vi "Export.vi"(9 "warehosue database table":string[](array[string]), 10 "Path":path, 11 "connection in":T4) -> (3 "connection out":T4)   [LabVIEW 2017]
uses:
  <vilib>/addons/database/Connection.llb/Conn ObjectReference.ctl
  Control/item colum type.ctl
  Control/Produce colum type.ctl
  <vilib>/Utility/miscctls.llb/LVPointTypeDef.ctl
  <vilib>/Utility/miscctls.llb/LVRowAndColumnUnsignedTypeDef.ctl
  Control/State machine.ctl
  Control/Label data.ctl
  <vilib>/addons/database/Connection.llb/DB Tools Open Connec (Path).vi
  <vilib>/addons/_office/excel.llb/Excel Get Data ([str]).vi
  <vilib>/addons/database/Connection.llb/Conn Execute.vi
  <vilib>/addons/database/Recordset.llb/Rec Fetch Recordset Data (R).vi
  <vilib>/addons/database/Recordset.llb/Rec Destroy - Connection.vi
  <vilib>/addons/database/_DB Variant To Data/Database Variant To Data.xnode
  <vilib>/Utility/NIReport.llb/NI_report.lvclass
  <vilib>/addons/_office/NI_ReportGenerationToolkit.lvlib
  <vilib>/addons/database/NI_Database_API.lvlib
  <vilib>/Utility/NIReport.llb/Excel/NI_Excel.lvclass
panel:
  out "output cluster":T1
  in  "produce_data":T1
  out "reference":refnum<vi>[](array[refnum])
  in  "Print Mode 2":bool=TRUE
  out "IQA":string
  out "stock":string
  in  "Print Mode":bool=TRUE
  in  "Print":bool
  in  "Item No.(F8)":i32
  in  "item_data":T2
  out "item_data_name":string[](array[string])
  out "item_data_ctr":refnum<vi>[](array[refnum])
  out "ECODE":string
  out "PRODUCE_data_ctr":refnum<vi>[](array[refnum])
  out "PRODUCE_data_name":string[](array[string])
  out "File data":string[][](array[string])
  in  "Import data":T3 {"produce Date" format="%<%d/%m/%Y>T"}
  in  "Lot Maker (F9)":string
  in  "Location (F5)":string
  in  "Maker Code (F4)":string
  in  "BUTTON_ADD":bool
  in  "Quantity (F10)":string
  in  "Lot Size (F6)":string
  in  "Unit (F7)":string
  in  "Item Code (F3)":string
  in  "Part No (F2)":string(combo)
  in  "Barcode (F1)":string
  in  "Offset":string="0"
  in  "Length":string="0"
  in  "Maker":string(combo)
  in  "Part Name":string(combo)
  in  "Product":string(combo)
  out "Produce Date":timestamp format="%<%d/%m/%Y>T"
  out "produce Code":string caption="Produce Code"
  out "Table":string[][](table)
  # "PRODUCE EXMPORT"
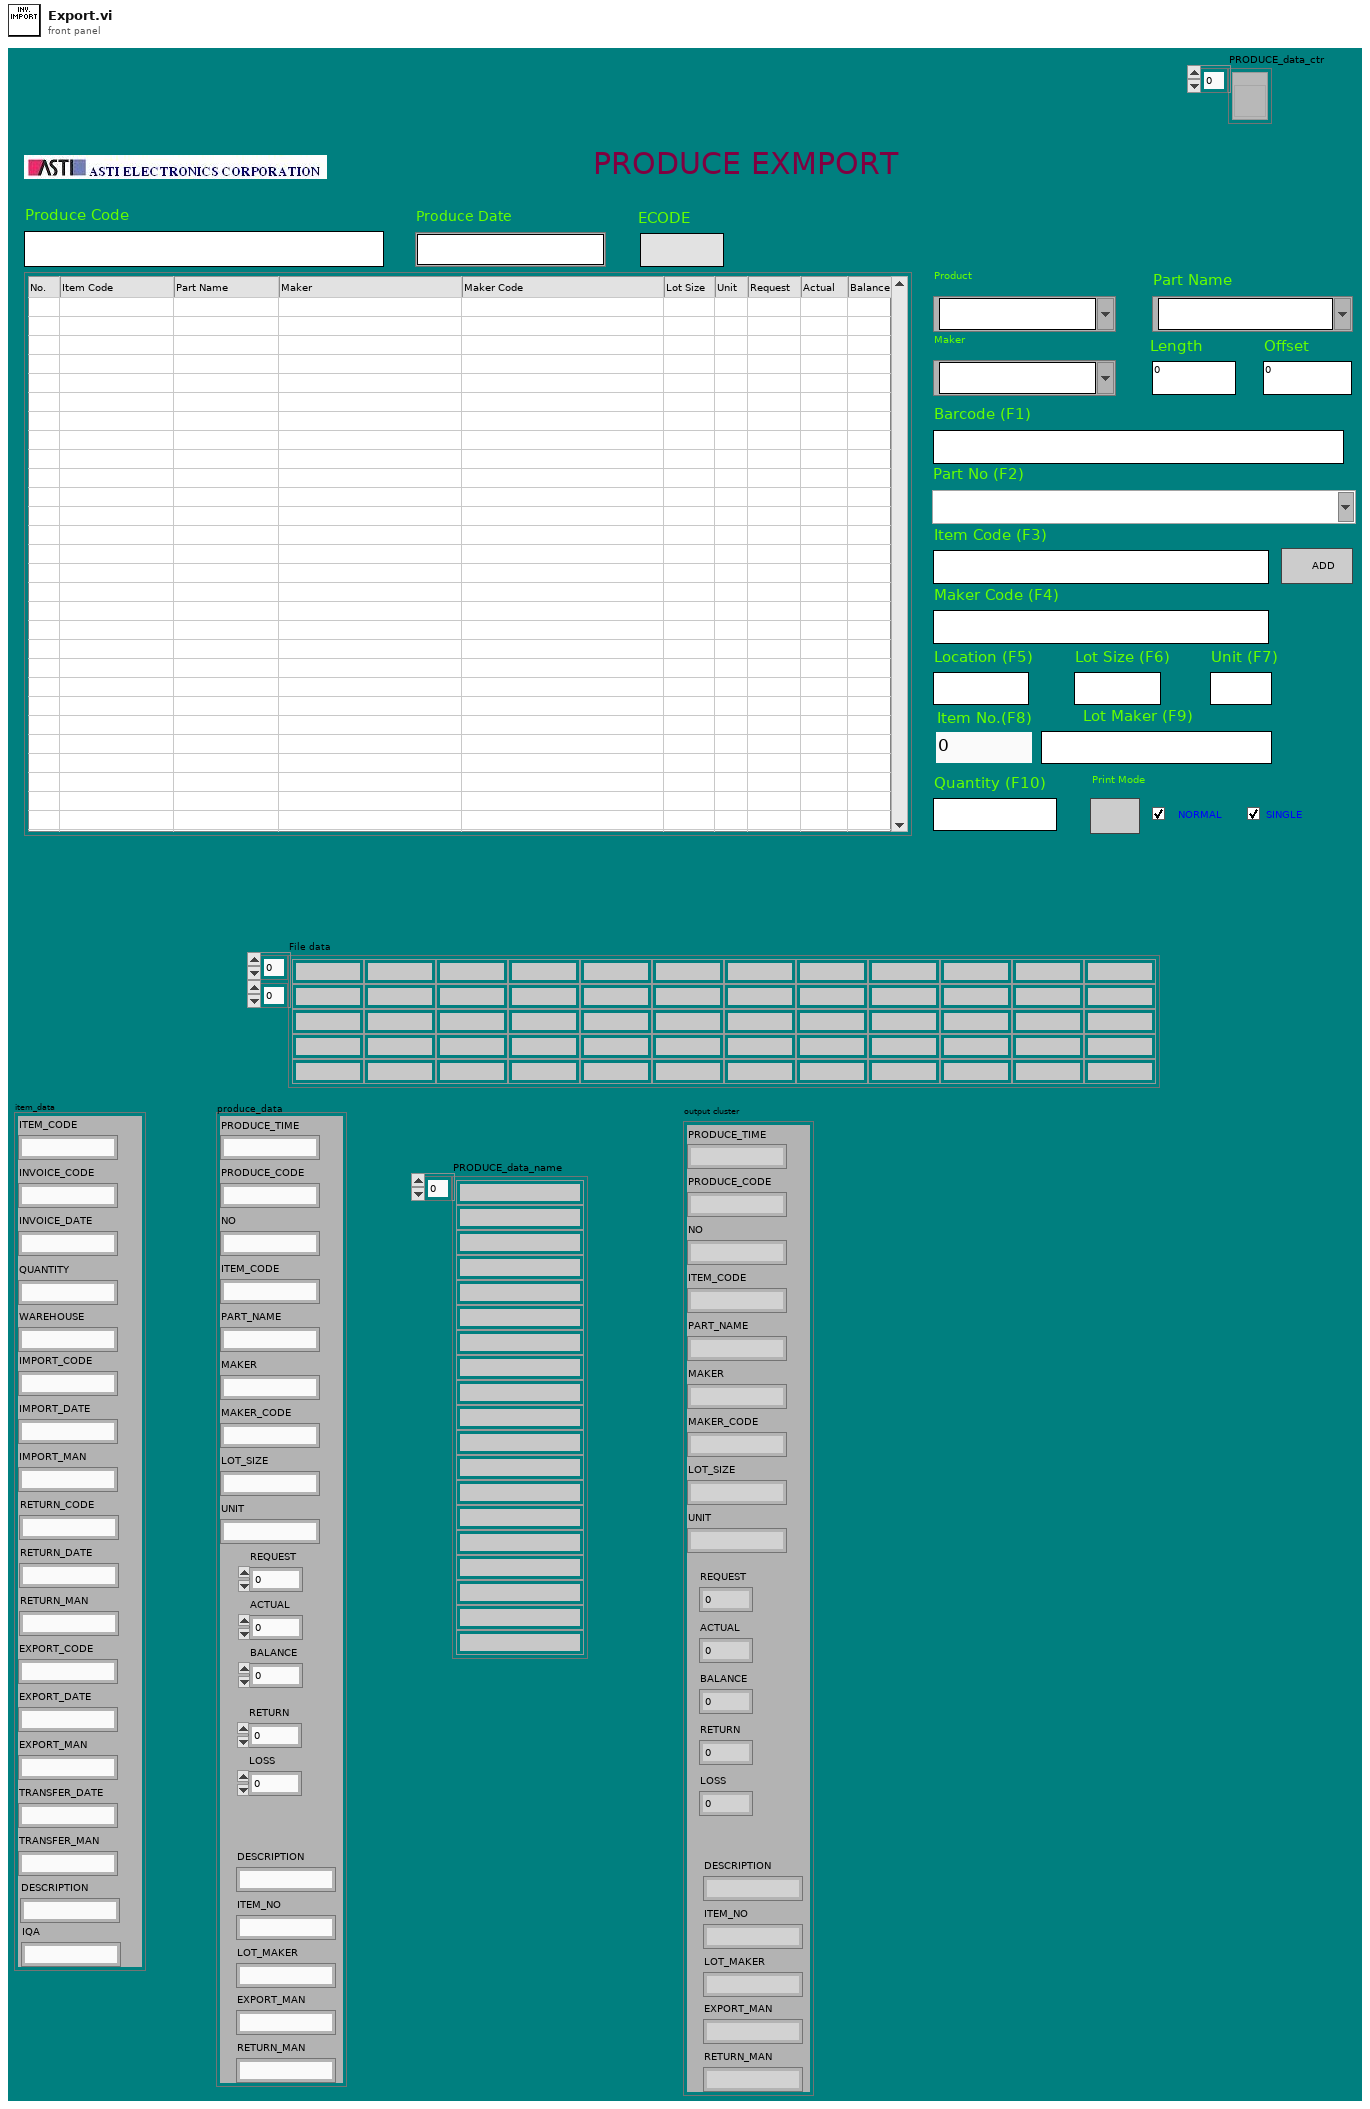
[diagram p1: front panel]
types:
  T1 = typedef "Produce colum type.ctl" = cluster{"PRODUCE_TIME":string, "PRODUCE_CODE":string, "NO":string, "ITEM_CODE":string, "PART_NAME":string, "MAKER":string, "MAKER_CODE":string, "LOT_SIZE":string, "UNIT":string, "REQUEST":u64, "ACTUAL":u64, "BALANCE":u64, "RETURN":u64, "LOSS":u64, "DESCRIPTION":string, "ITEM_NO":string, "LOT_MAKER":string, "EXPORT_MAN":string, "RETURN_MAN":string}
  T2 = typedef "item colum type.ctl" = cluster{"ITEM_CODE":string, "INVOICE_CODE":string, "INVOICE_DATE":string, "QUANTITY":string, "IMPORT_CODE":string, "IMPORT_DATE":string, "IMPORT_MAN":string, "RETURN_CODE":string, "RETURN_DATE":string, "RETURN_MAN":string, "EXPORT_CODE":string, "EXPORT_DATE":string, "EXPORT_MAN":string, "TRANSFER_DATE":string, "TRANSFER_MAN":string, "DESCRIPTION":string, "IQA":string, "WAREHOUSE":string}
  T3 = cluster{"produce Code":string, "produce Date":timestamp, "Import data":string[][]}
  T4 = typedef "NI_Database_API.lvlib/Conn ObjectReference.ctl" = refnum<k1>
  T5 = typedef "State machine.ctl" = enum16{"Licence check", "Initial", "Log in", "Creat Config file", "Network setting", "Creat database 1", "Creat database 2", "Creat database 3", "Transfer", "Begin", "Exit"}
  T6 = typedef "LVRowAndColumnUnsignedTypeDef.ctl" = cluster{"Row":u32, "Column":u32}
  T7 = typedef "LVPointTypeDef.ctl" = cluster{"Horizontal":i16, "Vertical":i16}
  T8 = enum8{"Enabled", "Disabled", "Disabled and Grayed Out"}
  T9 = enum16{"Standard Report", "HTML", "Word", "Excel"}
  T10 = enum16{"maximized", "minimized", "normal", "no change"}
  T11 = typedef "Label data.ctl" = cluster{"Item Code":string, "ECode":string, "Part No.":string, "Maker":string, "Quantity":string, "Location":string, "Product":string, "Invoice No":string, "Invoice Date":string, "Lot maker":string, "Item No":string, "Unit":string}
  T12 = typedef "NI_Database_API.lvlib/Rec ObjectReference.ctl" = refnum<k1>
  T13 = cluster{"data[0]":string, "data[1]":string, "data[2]":string, "data[3]":string, "data[4]":string, "data[5]":string, "data[6]":string, "data[7]":string, "data[8]":string, "data[9]":string}
  T14 = cluster{"data[0]":string, "data[1]":string, "data[2]":string, "data[3]":string, "data[4]":string, "data[5]":string, "data[6]":string, "data[7]":string, "data[8]":string, "data[9]":string}[]
  T15 = cluster{"date/time string":string, "produce Code":string}
  T16 = cluster{"Product":string, "Item Code (F3)":string, "Part Name":string, "Maker":string, "Maker Code (F4)":string, "Lot Size (F6)":string, "Unit (F7)":string, string, string, "Location (F5)":string}
  T17 = cluster{"Quantity (F10)":string, "ECODE":string, "produce Code":string, "Item Code (F3)":string, "Lot Maker (F9)":string, "stock":string, "IQA":string, string}
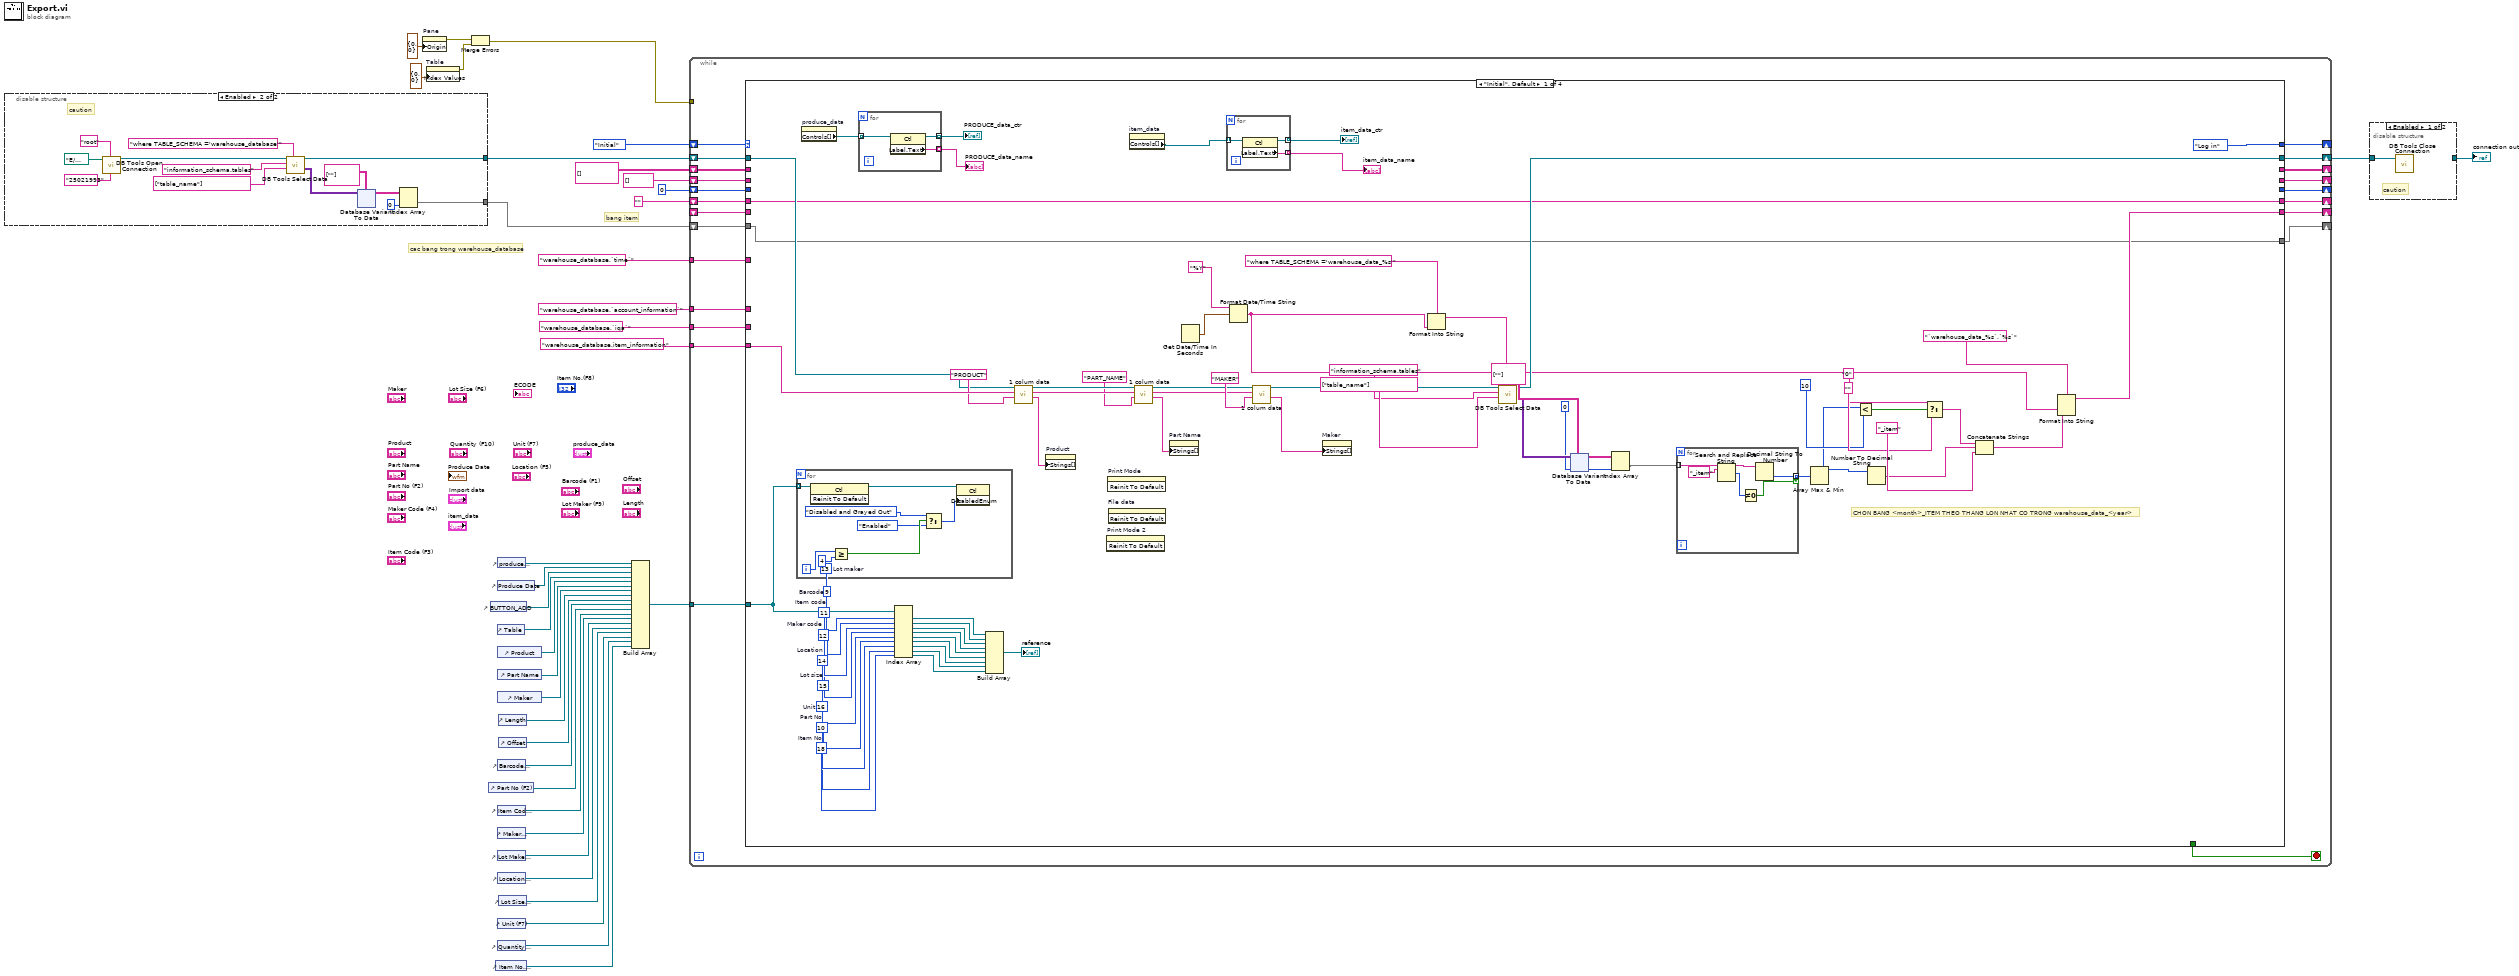
[diagram p0: block diagram]
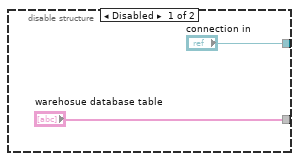
[diagram p3: hidden frame]
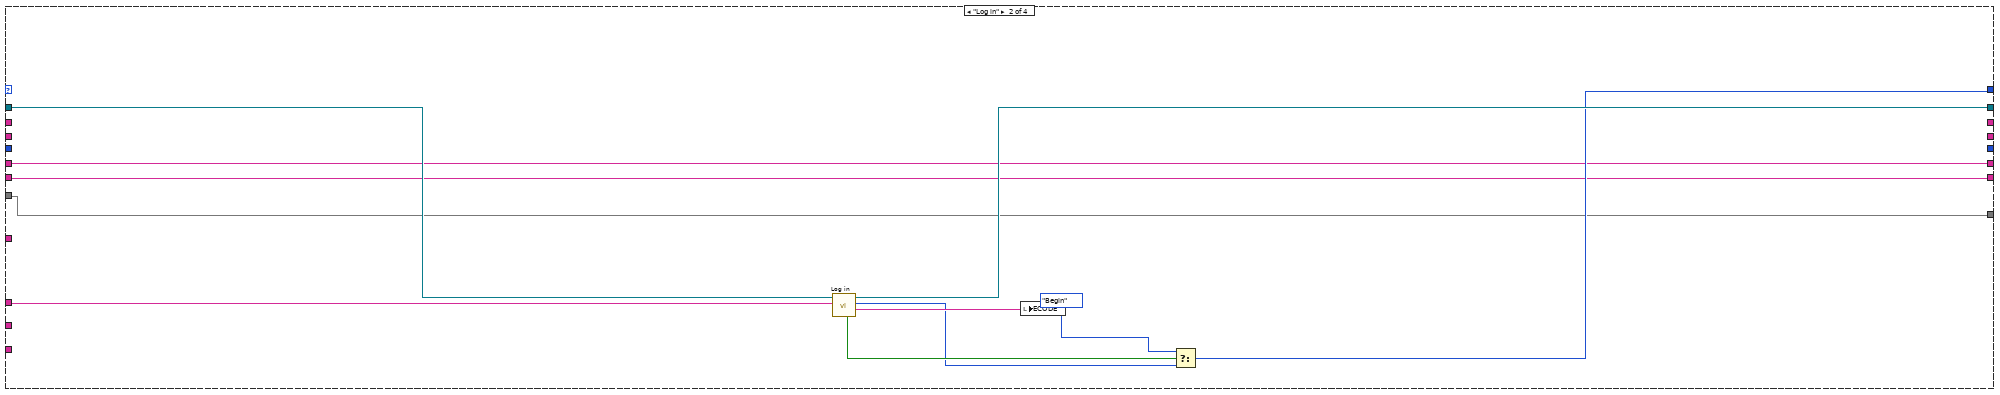
[diagram p4: hidden frame]
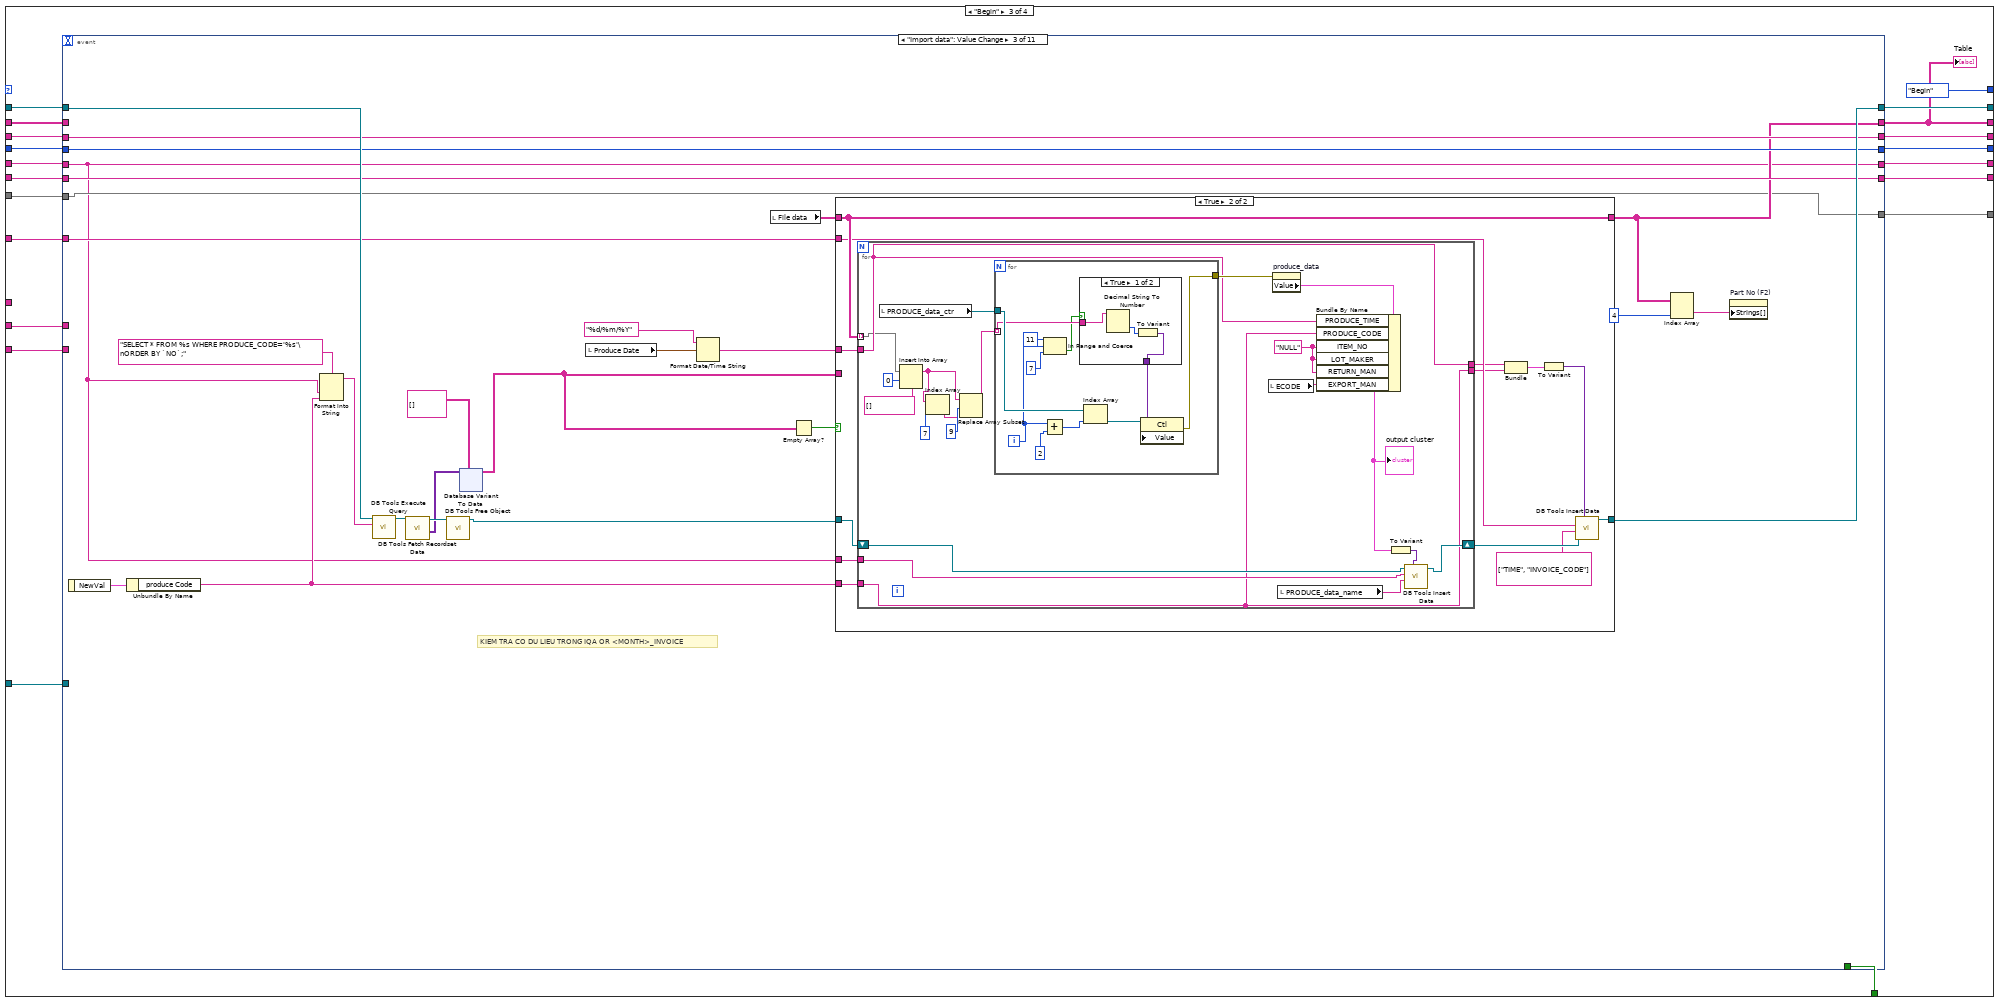
[diagram p5: hidden frame]
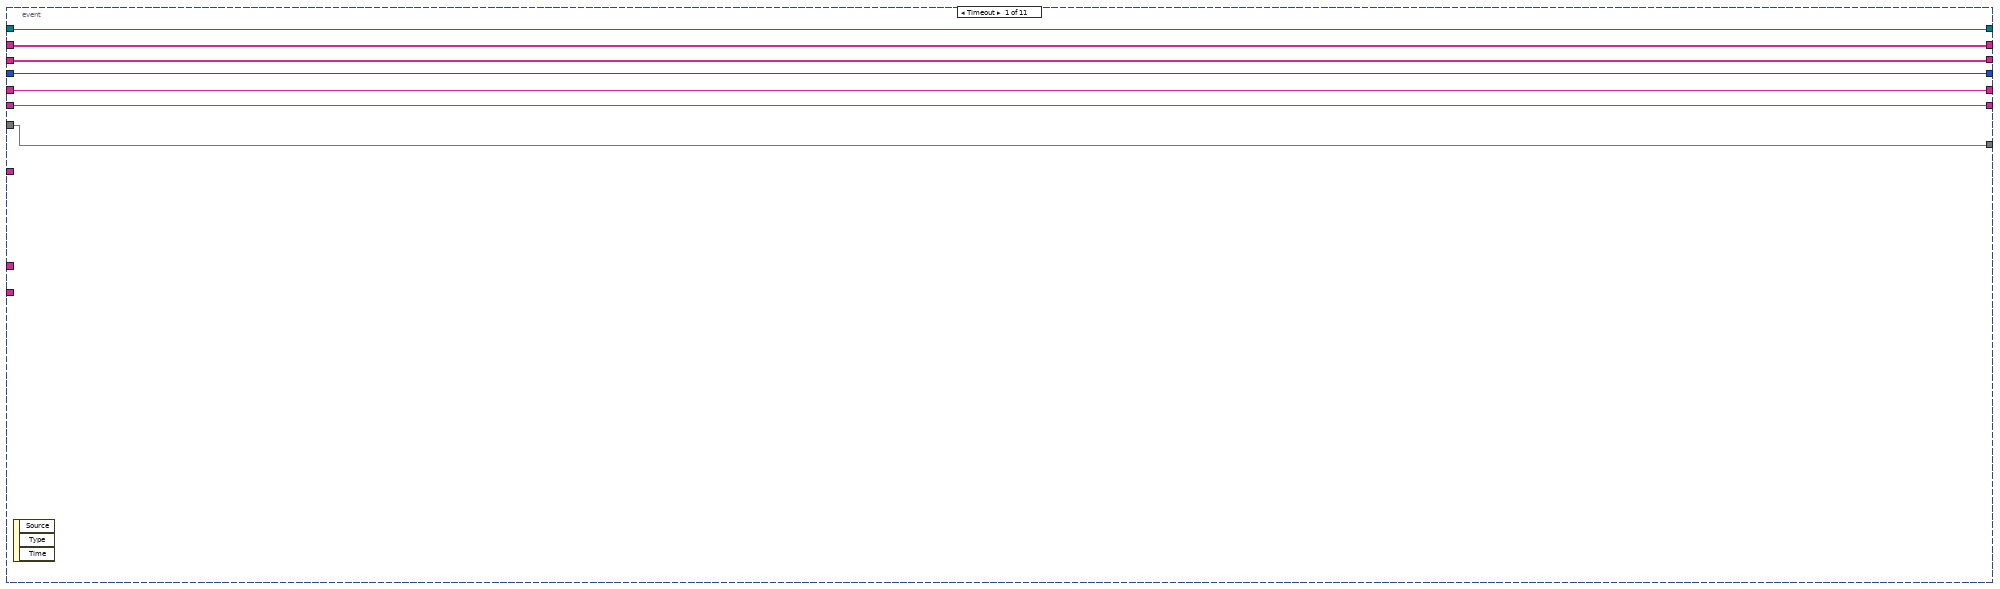
[diagram p6: hidden frame]
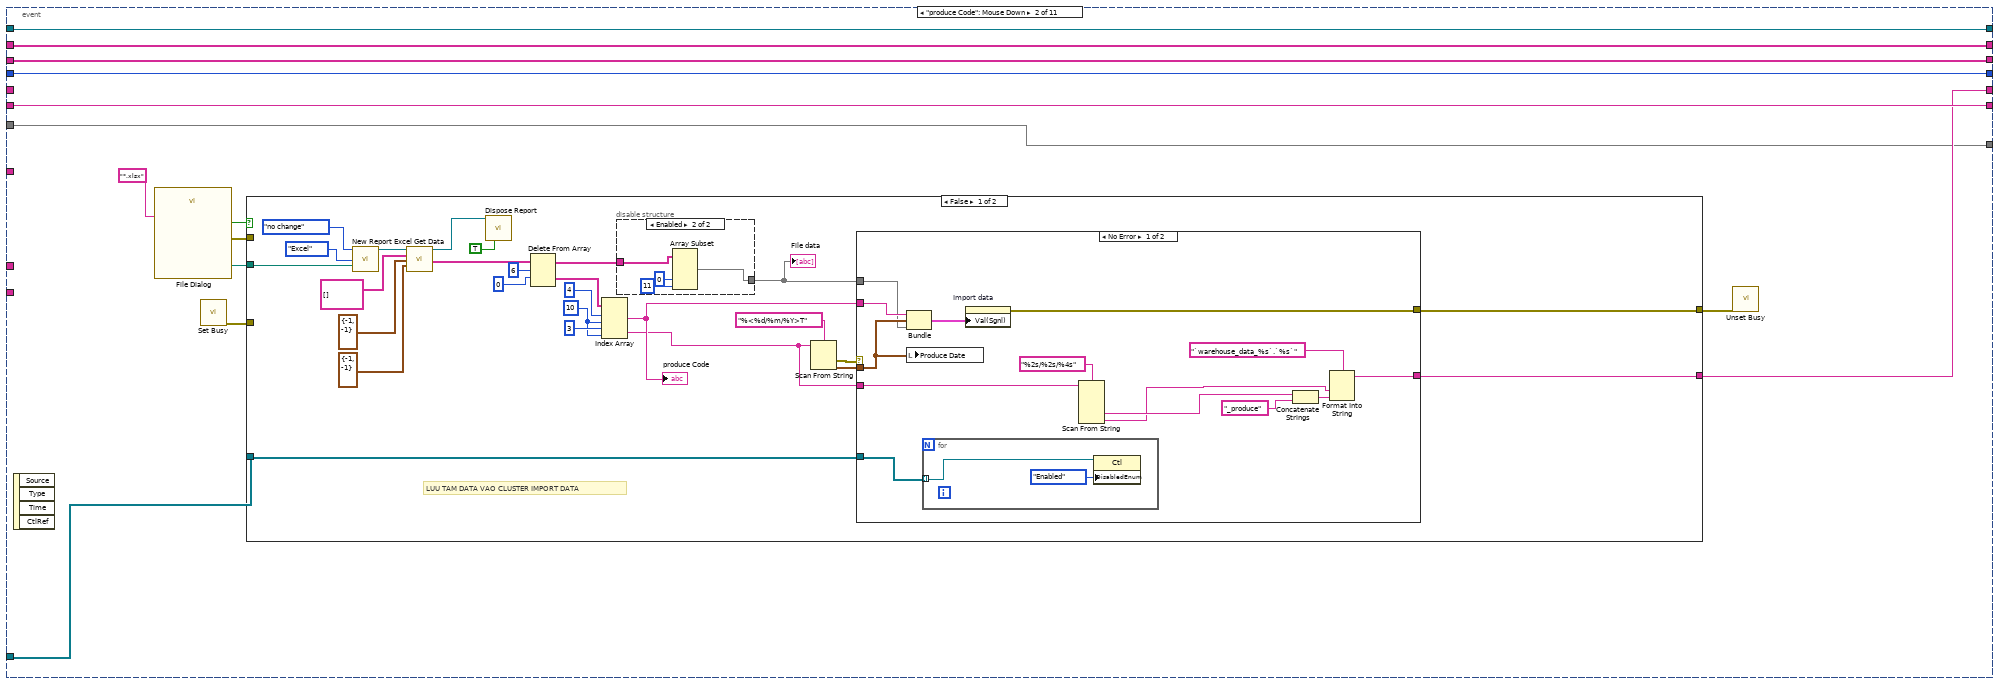
[diagram p7: hidden frame]
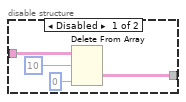
[diagram p8: hidden frame]
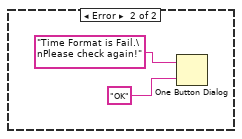
[diagram p9: hidden frame]
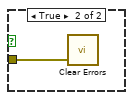
[diagram p10: hidden frame]
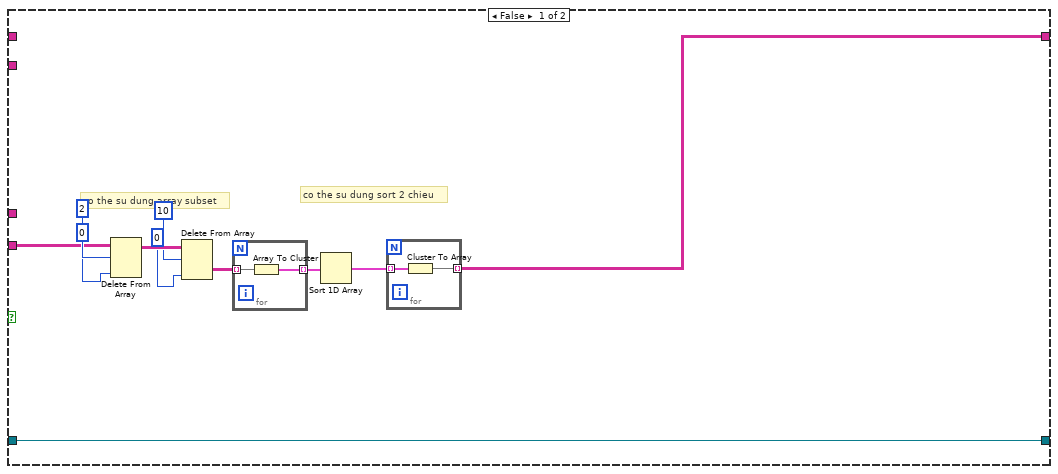
[diagram p11: hidden frame]
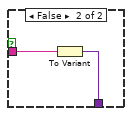
[diagram p12: hidden frame]
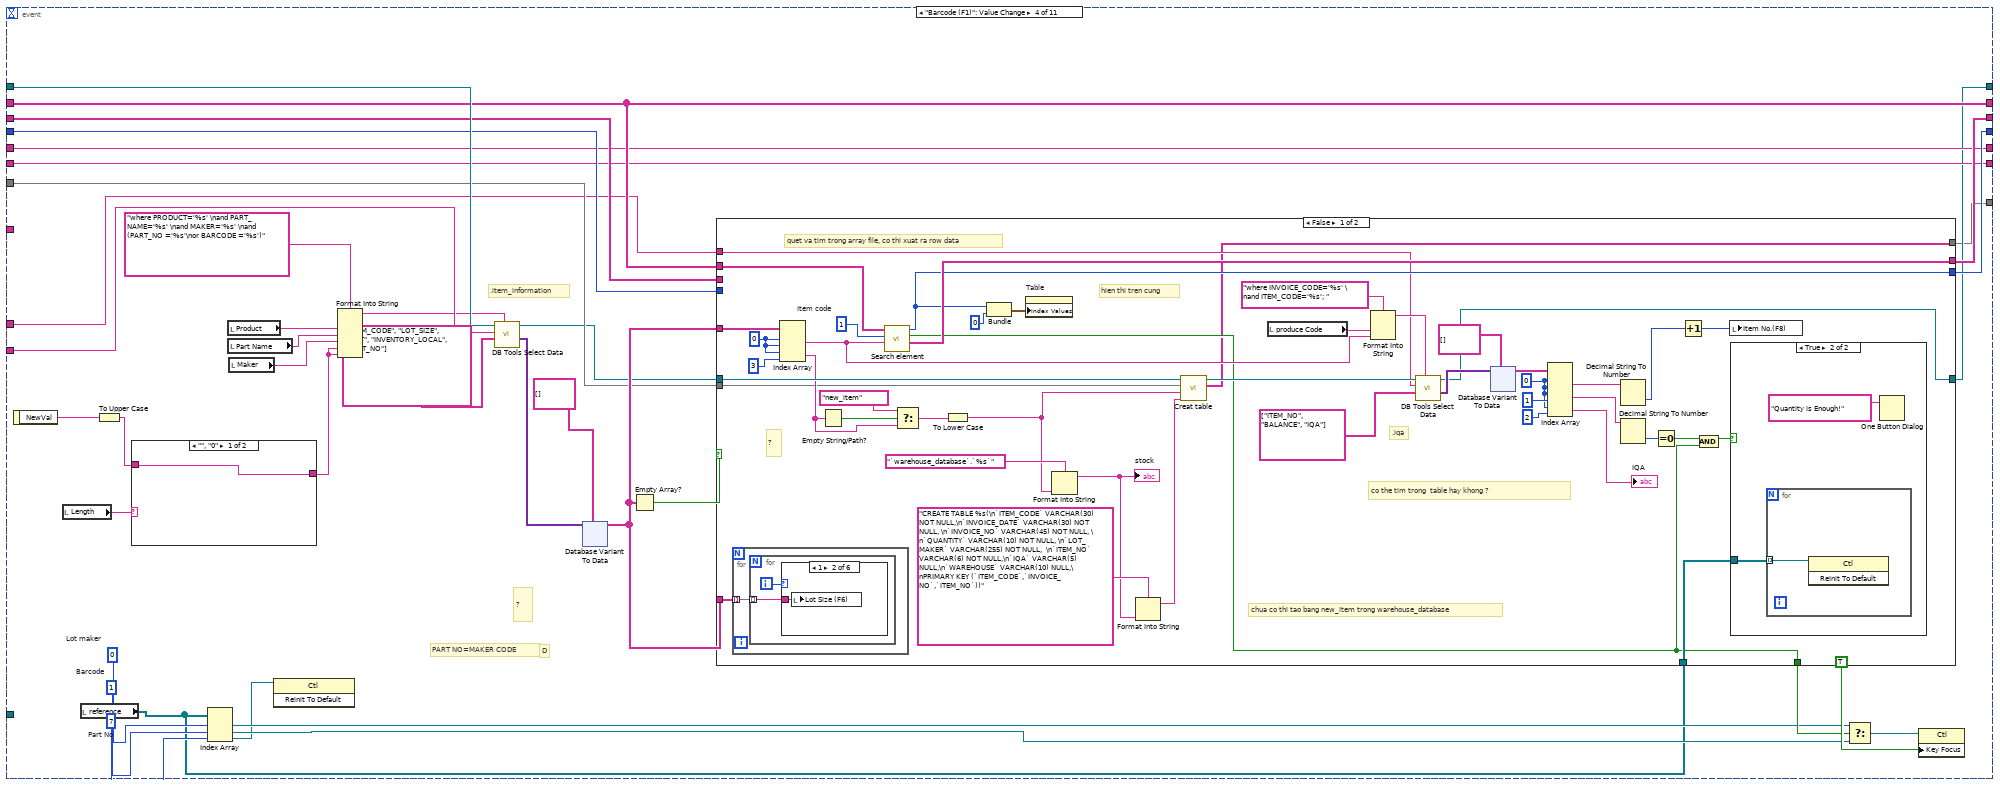
[diagram p13: hidden frame]
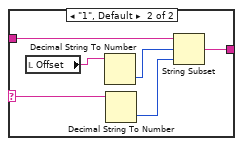
[diagram p14: hidden frame]
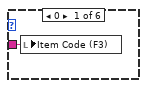
[diagram p16: hidden frame]
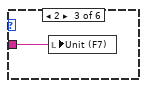
[diagram p17: hidden frame]
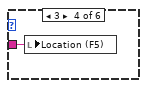
[diagram p18: hidden frame]
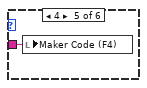
[diagram p19: hidden frame]
diagram:
  # "bang item"
  # "cac bang trong warehouse_database"
  n1 = disable-structure shown="Enabled" {
    disable-tunnel: ["connection in" w42] -> w16
    disable-tunnel: ["warehosue database table" w41] -> w3
    frame Disabled {
    }
    frame Enabled {
      # "caution"
      n2 = call-poly <vilib>:"DB Tools Open Connection.vi"("password"="25021993", "userID"="root", "connection information"=path "E:/PROJECT WORKING/23. WAREHOUSE/New Storage Management 2018/Setting/local.dsn") -> ("connection reference"=w43:T4)  [unwired: 5 in, 1 out]
      n3 = call <vilib>:"DB Tools Select Data.vi"("condition"="where TABLE_SCHEMA ='warehouse_database'", "columns"=string[] ["table_name"], "table"="information_schema.tables", "connection reference"=w43) -> ("data"=w46:variant[][], "connection reference out"=w42:T4)  [unwired: 2 in, 1 out]
      n4 = xnode "Database Variant To Data"("database variant"=w46, "type"=string[][] [[""]] ("columns")) -> ("data"=w48:string[][])  [unwired: 1 in, 1 out]
      n5 = Index Array(array=w48, index (col)=0 ("disabled index (col)")) -> (element=w41:string[])  [unwired: 1 in]
    }
  }
  n6 = property on="Pane" class="Pane"("Origin"=T7 {"Horizontal"=0, "Vertical"=0}) -> (error out=w36:errorcluster)  [unwired: 2 in, 1 out]
  n7 = property on="Table" class="Tbl (strict)"("Index Values"=T6 {"Row"=0, "Column"=0}) -> (error out=w35:errorcluster)  [unwired: 2 in, 1 out]
  n8 = Merge Errors(w36, w35) -> (w12:errorcluster)
  n9 = control-ref of="Part No (F2)"() -> (w25:refnum<vi>)
  n10 = control-ref of="BUTTON_ADD"() -> (w1:refnum<vi>)
  n11 = control-ref of="Item No.(F8)"() -> (w2:refnum<vi>)
  n12 = control-ref of="produce Code"() -> (w34:refnum<vi>)
  n13 = control-ref of="Produce Date"() -> (w33:refnum<vi>)
  n14 = control-ref of="Table"() -> (w32:refnum<vi>)
  n15 = control-ref of="Product"() -> (w31:refnum<vi>)
  n16 = control-ref of="Part Name"() -> (w30:refnum<vi>)
  n17 = control-ref of="Maker"() -> (w29:refnum<vi>)
  n18 = control-ref of="Barcode (F1)"() -> (w26:refnum<vi>)
  n19 = control-ref of="Item Code (F3)"() -> (w24:refnum<vi>)
  n20 = control-ref of="Maker Code (F4)"() -> (w23:refnum<vi>)
  n21 = control-ref of="Lot Maker (F9)"() -> (w22:refnum<vi>)
  n22 = control-ref of="Location (F5)"() -> (w21:refnum<vi>)
  n23 = control-ref of="Unit (F7)"() -> (w19:refnum<vi>)
  n24 = control-ref of="Quantity (F10)"() -> (w13:refnum<vi>)
  n25 = control-ref of="Length"() -> (w28:refnum<vi>)
  n26 = control-ref of="Offset"() -> (w27:refnum<vi>)
  n27 = control-ref of="Lot Size (F6)"() -> (w20:refnum<vi>)
  n28 = Build Array(w34, w33, w1, w32, w31, w30, w29, w28, w27, w26, w25, w24, w23, w22, w21, w20, w19, w13, w2) -> (w18:refnum<vi>[])
  n29 = while {
    tunnel: w18 -> [w117]
    shift-right: [w116] -> _
    shift-left: State_machine."Initial" ("Enum") -> [w118]
    shift-right: [w114] -> w15
    shift-left: w16 -> [w115]
    tunnel: w12 -> [_]
    shift-right: [w113] -> _
    shift-left: string[][] [] ("File data") -> [w112]
    tunnel: "warehouse_database.item_information" -> [w110]
    shift-right: [w109] -> _
    shift-left: string[] [] ("row data") -> [w108]
    shift-right: [w107] -> _
    shift-left: 0 ("index") -> [w106]
    tunnel: "warehouse_database.`iqa`" -> [w105]
    tunnel: "warehouse_database.`account_information`" -> [w103]
    tunnel: "warehouse_database.`time`" -> [w102]
    shift-right: [w101] -> _
    shift-left: "" -> [w111]
    shift-right: [w100] -> _
    shift-left: _ -> [w104]
    shift-right: [w98] -> _
    shift-left: w3 -> [w99]
    stop <- w119 stop-if-true
    n30 = case shown="\"Initial\", Default" w118 {
      selector: w118 -> [_ _ _ w1199]
      tunnel: [_ _ w281 TRUE ("T button?")] -> w119
      tunnel: w117 -> [w124 _ w275 _]
      tunnel: [State_machine."Log in" ("Enum") w254 State_machine."Begin" ("Enum") w1199] -> w116
      tunnel: w115 -> [w173 w261 w279 w1200]
      tunnel: [w163 w260 w278 w1200] -> w114
      tunnel: [_ _ w277 _] -> w113
      tunnel: w112 -> [_ _ w276 _]
      tunnel: w111 -> [w149 w252 w274 _]
      tunnel: w110 -> [w182 _ w273 _]
      tunnel: [_ _ w272 _] -> w109
      tunnel: w108 -> [_ _ w271 _]
      tunnel: [_ _ w270 _] -> w107
      tunnel: w106 -> [_ _ w269 _]
      tunnel: w105 -> [_ _ w268 _]
      tunnel: w104 -> [_ w253 w267 w1198]
      tunnel: w103 -> [_ w259 _ _]
      tunnel: w102 -> [_ _ w266 _]
      tunnel: [w149 w252 w264 _] -> w101
      tunnel: [w150 w253 w265 w1198] -> w100
      tunnel: w99 -> [w122 w251 w263 w1197]
      tunnel: [w122 w251 w262 w1197] -> w98
      frame "Initial", Default {
        w128 = 18  # Item No
        w129 = 10  # Part No
        w136 = 16  # Unit
        w137 = 15  # Lot size
        w138 = 14  # Location
        w139 = 12  # Maker code
        w140 = 11  # Item code
        w141 = 9  # Barcode
        w142 = 13  # Lot maker
        # "CHON BANG <month>_ITEM THEO THANG LON NHAT CO TRONG warehouse_data_<year>"
        n31 = for {
          tunnel: w124 -> [w250] mode=indexing
          i -> [w249]
          n32 = invoke class="Ctl" method="Reinit To Default"(reference=w250) -> (reference out=w247:refnum<vi>)  [unwired: 2 in, 2 out]
          n33 = Greater Or Equal?(x=w249, y=4) -> (x >= y?=w246:bool)
          n34 = Select(t=T8."Disabled and Grayed Out" ("Disabled"), s=w246, f=T8."Enabled" ("Disabled")) -> (s? t:f=w243:T8)
          n35 = property class="Ctl"(reference=w247, "DisabledEnum"=w243) -> ()  [unwired: 1 in, 2 out]
        }
        n36 = property on="produce_data" class="Clust (strict)"() -> ("Controls[]"=w121:refnum<vi>[])  [unwired: 2 in, 2 out]
        n37 = for {
          tunnel: w121 -> [w242] mode=indexing
          tunnel: [w241] -> w185 mode=indexing
          tunnel: [w240] -> w184 mode=indexing
          n38 = property class="Ctl"(reference=w242) -> (reference out=w240:refnum<vi>, "Label.Text"=w241:string)  [unwired: 1 in, 1 out]
        }
        "PRODUCE_data_name" <- w185
        "PRODUCE_data_ctr" <- w184
        n39 = Index Array(array=w124, index #1=w142, index #2=w141, index #3=w140, index #4=w139, index #5=w138, index #6=w137, index #7=w136, index #8=w129, index #9=w128) -> (element #1=w130:refnum<vi>, element #2=w125:refnum<vi>, element #3=w135:refnum<vi>, element #4=w134:refnum<vi>, element #5=w133:refnum<vi>, element #6=w132:refnum<vi>, element #7=w131:refnum<vi>, element #8=w126:refnum<vi>, element #9=w127:refnum<vi>)
        n40 = Build Array(w130, w125, w135, w134, w133, w132, w131, w126, w127) -> (→"reference":refnum<vi>[])
        n41 = call "1 colum data.vi"("column"="PRODUCT", "table"=w182, "Refnum in"=w173) -> ("data"=w180:string[], "table"=w179:string, "Refnum out"=w183:T4)  [unwired: 6 in]
        n42 = property on="Product" class="CmbBox"("Strings[]"=w180) -> ()  [unwired: 2 in, 2 out]
        n43 = invoke on="Print Mode 2" class="Bool (strict)" method="Reinit To Default"() -> ()  [unwired: 3 in, 3 out]
        n44 = invoke on="Print Mode" class="Bool (strict)" method="Reinit To Default"() -> ()  [unwired: 3 in, 3 out]
        n45 = invoke on="File data" class="Arr (strict)" method="Reinit To Default"() -> ()  [unwired: 3 in, 3 out]
        n46 = property on="item_data" class="Clust (strict)"() -> ("Controls[]"=w120:refnum<vi>[])  [unwired: 2 in, 2 out]
        n47 = call "1 colum data.vi"("column"="PART_NAME", "table"=w179, "Refnum in"=w183) -> ("data"=w177:string[], "table"=w172:string, "Refnum out"=w174:T4)  [unwired: 6 in]
        n48 = property on="Part Name" class="CmbBox"("Strings[]"=w177) -> ()  [unwired: 2 in, 2 out]
        n49 = Get Date/Time In Seconds() -> (seconds since 1Jan1904=w148:timestamp)
        n50 = for {
          tunnel: w120 -> [w239] mode=indexing
          tunnel: [w238] -> w170 mode=indexing
          tunnel: [w237] -> w171 mode=indexing
          n51 = property class="Ctl"(reference=w239) -> (reference out=w237:refnum<vi>, "Label.Text"=w238:string)  [unwired: 1 in, 1 out]
        }
        "item_data_name" <- w170
        "item_data_ctr" <- w171
        n52 = Format Date/Time String(time format string (%c)="%Y", seconds (now)=w148) -> (date/time string=w143:string)  [unwired: 1 in]
        n53 = call "1 colum data.vi"("column"="MAKER", "table"=w172, "Refnum in"=w174) -> ("data"=w176:string[], "Refnum out"=w164:T4)  [unwired: 6 in, 1 out]
        n54 = property on="Maker" class="CmbBox"("Strings[]"=w176) -> ()  [unwired: 2 in, 2 out]
        n55 = Format Into String(format string="where TABLE_SCHEMA ='warehouse_data_%s'" ("condition"), w143) -> (resulting string=w145:string)  [unwired: 2 in, 1 out]
        n56 = call <vilib>:"DB Tools Select Data.vi"("condition"=w145, "columns"=string[] ["table_name"], "table"="information_schema.tables", "connection reference"=w164) -> ("data"=w167:variant[][], "connection reference out"=w163:T4)  [unwired: 2 in, 1 out]
        n57 = xnode "Database Variant To Data"("database variant"=w167, "type"=string[][] [[""]] ("columns")) -> ("data"=w169:string[][])  [unwired: 1 in, 1 out]
        n58 = Index Array(array=w169, index (col)=0 ("disabled index (col)")) -> (element=w152:string[])  [unwired: 1 in]
        n59 = for {
          tunnel: w152 -> [w192] mode=indexing
          tunnel: [w187] -> w153 mode=indexing if=w189
          n60 = Search and Replace String(input string=w192, search string="_item") -> (result string=w188:string, number of replacements=w190:i32)  [unwired: 6 in, 2 out]
          n61 = Not Equal To 0?(x=w190) -> (x != 0?=w189:bool)
          n62 = Decimal String To Number(string=w188) -> (number=w187:i32)  [unwired: 2 in, 1 out]
        }
        n63 = Array Max & Min(array=w153) -> (max value=w154:i32)  [unwired: 3 out]
        n64 = Less?(x=w154, y=10) -> (x < y?=w156:bool)
        n65 = Number To Decimal String(number=w154) -> (decimal integer string=w160:string)  [unwired: 1 in]
        n66 = Select(t="0", s=w156, f="" ("t")) -> (s? t:f=w159:string)
        n67 = Concatenate Strings(w159, w160, "_item" ("string")) -> (w144:string)
        n68 = Format Into String(format string="`warehouse_data_%s`.`%s`", w143, w144) -> (resulting string=w150:string)  [unwired: 2 in, 1 out]
      }
      frame "Log in" {
        n69 = call "Log in.vi"("String in"=w259, "Refnum in"=w261) -> ("String out"=w258:string, "Enum"=w256:T5, "Refnum out"=w260:T4, "T/F"=w257:bool)  [unwired: 5 in, 1 out]
        n70 = local write "ECODE"(w258) -> ()
        n71 = Select(t=State_machine."Begin", s=w257, f=w256) -> (s? t:f=w254:T5)
      }
      frame "Begin" {
        n72 = event shown="[2] \"Import data\": Value Change" {
          selector: _ -> [_ _ _ _ _ _ _ _ _ _ _]
          dyn-events: _ -> [_ _ _ _ _ _ _ _ _ _ _]
          timeout: _ -> [_ _ _ _ _ _ _ _ _ _ _]
          tunnel: [_ _ _ _ _ _ _ _ _ _ w1195] -> w281
          tunnel: w279 -> [w288 w302 w381 w528 w693 w730 w902 w1005 w1103 w1183 w1194]
          tunnel: [w288 w302 w373 w498 w693 w703 w906 w1003 w1102 w1183 w1194] -> w278
          tunnel: [w287 w300 w362 w510 w692 w714 w905 w1001 w1101 w1182 w1193] -> w277
          tunnel: w276 -> [w287 w300 _ w510 w692 w714 w905 w1002 w1101 w1182 w1193]
          tunnel: w275 -> [_ w301 _ _ _ _ _ w1006 w1100 w1187 _]
          tunnel: w274 -> [w284 _ w356 w504 w689 w708 w884 w1004 w1097 w1179 w1190]
          tunnel: w273 -> [_ _ _ w514 _ w718 w900 _ w1093 _ _]
          tunnel: [w286 w299 w372 w508 w691 w712 w904 w1000 w1099 w1181 w1192] -> w272
          tunnel: w271 -> [w286 w299 w372 w507 w691 w711 w904 w1000 w1099 w1181 w1192]
          tunnel: [w285 w298 w371 w506 w690 w710 w903 w999 w1098 w1180 w1191] -> w270
          tunnel: w269 -> [w285 w298 w371 w505 w690 w709 w903 w999 w1098 w1180 w1191]
          tunnel: w268 -> [_ _ _ w499 _ w704 _ w998 _ _ _]
          tunnel: w267 -> [w283 w297 w363 w503 w688 w707 w883 w984 w1096 w1178 w1189]
          tunnel: w266 -> [_ _ w366 _ _ _ _ _ _ _ _]
          tunnel: [w283 w297 w363 w503 w688 w707 w883 w984 w1096 w1178 w1189] -> w265
          tunnel: [w284 w296 w356 w504 w689 w708 w884 w1004 w1097 w1179 w1190] -> w264
          tunnel: w263 -> [w282 w289 w359 w502 w687 w706 w882 w983 w1092 w1176 w1188]
          tunnel: [w282 w289 w359 w491 w687 w696 w882 w983 w1092 w1176 w1188] -> w262
          event Timeout {
            n73 = event-data() -> ()  [unwired: 1 in, 3 out]
          }
          event "produce Code": Mouse Down {
            n74 = event-data() -> ()  [unwired: 1 in, 4 out]
            n75 = call "File Dialog"("pattern (all files)"="*.xlsx") -> ("selected path"=w292:path, "cancelled"=w294:bool, "error out"=w293:errorcluster)  [unwired: 11 in, 1 out]
            n76 = call <vilib>:"Set Busy.vi"() -> ("error out"=w291:errorcluster)  [unwired: 10 in, 1 out]
            n77 = case shown="False" w294 {
              tunnel: w293 -> [_ w355]
              tunnel: w292 -> [w328 _]
              tunnel: w291 -> [_ _]
              tunnel: [w306 _] -> w290
              tunnel: w301 -> [w307 _]
              tunnel: [w304 _] -> w296
              frame False {
                w303 = 10 ("disabled index (col)")
                # "LUU TAM DATA VAO CLUSTER IMPORT DATA"
                n78 = call <vilib>:"New Report.vi"("window state (normal)"=T10."no change", "report type"=T9."Excel", "template (empty)"=w328) -> ("report out"=w325:refnum<class "NI_report.lvclass">)  [unwired: 11 in, 1 out]
                n79 = call-poly <vilib>:"Excel Get Data.vi"("report in"=w325, "data type"=string[][] [], "start (-1, -1)"=cluster{"start row":i32, "start column":i32} {"start row"=-1, "start column"=-1} ("start (0, 0)"), "end (-1, -1)"=cluster{"start row":i32, "start column":i32} {"start row"=-1, "start column"=-1} ("start (0, 0)")) -> ("report out"=w324:refnum<class "NI_report.lvclass">, "data"=w319:string[][])  [unwired: 9 in, 1 out]
                n80 = call-dynamic "Dispose Report.vi"("report in"=w324, "close report? (T)"=TRUE) -> ()  [unwired: 13 in, 1 out]
                n81 = Delete From Array(array=w319, length=6, index (row)=0 ("length")) -> (deleted portion=w316:string[][], array with subset deleted=w309:string[][])  [unwired: 1 in]
                n82 = Index Array(array=w316, index (row) #1=4 ("index (row)"), index (col) #1=w303, index (row) #2=3 ("disabled index (row)"), index (col) #2=w303) -> (element #1=w310:string, element #2=w305:string)
                "produce Code" <- w310
                n83 = disable-structure shown="Enabled" {
                  disable-tunnel: w309 -> [w332 w336]
                  disable-tunnel: [w329 w333] -> w308
                  frame Disabled {
                    n84 = Delete From Array "Delete From Array"(array=w332, length=10, index (col)=0 ("disabled index (col)")) -> (deleted portion=w329:string[][])  [unwired: 1 in, 1 out]
                  }
                  frame Enabled {
                    n85 = Array Subset(array=w336, index (col)=0 ("index"), length (col)=11 ("length")) -> (w333:string[][])  [unwired: 2 in]
                  }
                }
                "File data" <- w308
                n86 = Scan From String(format string="%<%d/%m/%Y>T", input string=w305) -> (error out=w312:errorcluster, output 1=w311:timestamp)  [unwired: 3 in, 2 out]
                n87 = case shown="No Error" w312 {
                  tunnel: w311 -> [w348 _]
                  tunnel: w308 -> [w347 _]
                  tunnel: w310 -> [w349 _]
                  tunnel: w307 -> [w345 _]
                  tunnel: [w346 _] -> w306
                  tunnel: w305 -> [w344 _]
                  tunnel: [w339 _] -> w304
                  frame No Error {
                    n88 = Bundle(w349, w348, w347) -> (w350:cluster{string, timestamp, string[][]})  [unwired: 1 in]
                    n89 = local write "Produce Date"(w348) -> ()
                    n90 = for {
                      tunnel: w345 -> [w352] mode=indexing
                      n91 = property class="Ctl"(reference=w352, "DisabledEnum"=T8."Enabled" ("Disabled")) -> ()  [unwired: 1 in, 2 out]
                    }
                    n92 = property on="Import data" class="Clust (strict)"("Val(Sgnl)"=w350) -> (error out=w346:errorcluster)  [unwired: 2 in, 1 out]
                    n93 = Scan From String(format string="%2s/%2s/%4s", input string=w344) -> (output 2=w340:string, output 3=w337:string)  [unwired: 6 in, 3 out]
                    n94 = Concatenate Strings(w340, "_produce" ("string")) -> (w338:string)
                    n95 = Format Into String(format string="`warehouse_data_%s`.`%s`", w337, w338) -> (resulting string=w339:string)  [unwired: 2 in, 1 out]
                  }
                  frame Error {
                    n96 = One Button Dialog(message="Time Format is Fail.\nPlease check again!", button name ("OK")="OK") -> ()  [unwired: 1 out]
                  }
                }
              }
              frame True {
                n97 = call <vilib>:"Clear Errors.vi"("error in (no error)"=w355) -> ()  [unwired: 5 in, 2 out]
              }
            }
            n98 = call <vilib>:"Unset Busy.vi"("error in (no error)"=w290) -> ()  [unwired: 10 in, 1 out]
          }
          event "Import data": Value Change {
            # "KIEM TRA CO DU LIEU TRONG IQA OR <MONTH>_INVOICE"
            n99 = event-data() -> ("NewVal"=w380:T3)  [unwired: 1 in]
            n100 = Unbundle By Name(w380) -> ("produce Code"=w364:string)
            n101 = Format Into String(format string="SELECT * FROM %s WHERE PRODUCE_CODE='%s'\nORDER BY `NO`;", w356, w364) -> (resulting string=w379:string)  [unwired: 2 in, 1 out]
            n102 = call-poly <vilib>:"DB Tools Execute Query.vi"("SQL query"=w379, "connection reference"=w381) -> ("recordset reference"=w378:T12)  [unwired: 6 in, 1 out]
            n103 = call-poly <vilib>:"DB Tools Fetch Recordset Data.vi"("recordset reference"=w378) -> ("recordset data"=w375:variant[][], "recordset reference out"=w377:T12)  [unwired: 4 in, 1 out]
            n104 = call-poly <vilib>:"DB Tools Free Object.vi"("recordset reference"=w377) -> ("connection reference"=w357:T4)  [unwired: 9 in, 1 out]
            n105 = xnode "Database Variant To Data"("database variant"=w375, "type"=string[][] []) -> ("data"=w358:string[][])  [unwired: 1 in, 1 out]
            n106 = local read "Produce Date"() -> (w370:timestamp)
            n107 = Format Date/Time String(time format string (%c)="%d/%m/%Y", seconds (now)=w370) -> (date/time string=w369:string)  [unwired: 1 in]
            n108 = local read "File data"() -> (w368:string[][])
            n109 = Empty Array?(array=w358) -> (empty?=w374:bool)
            n110 = case shown="True" w374 {
              tunnel: [w383 w406] -> w362
              tunnel: w357 -> [w387 w409]
              tunnel: [w387 w403] -> w373
              tunnel: w364 -> [_ w408]
              tunnel: w358 -> [w382 _]
              tunnel: w369 -> [_ w407]
              tunnel: w368 -> [_ w406]
              tunnel: w356 -> [_ w405]
              tunnel: w366 -> [_ w402]
              frame False {
                # "co the su dung sort 2 chieu"
                # "co the su dung array subset"
                n111 = Delete From Array "Delete From Array"(array=w382, length=2, index (col)=0 ("disabled index (col)")) -> (array with subset deleted=w390:string[][])  [unwired: 1 in, 1 out]
                n112 = Delete From Array(array=w390, length=10, index (col)=0 ("disabled index (col)")) -> (deleted portion=w386:string[][])  [unwired: 1 in, 1 out]
                n113 = for {
                  tunnel: w386 -> [w396] mode=indexing
                  tunnel: [w395] -> w385 mode=indexing
                  n114 = Array To Cluster(array=w396) -> (cluster=w395:T13)
                }
                n115 = Sort 1D Array(array=w385) -> (sorted array=w384:T14)
                n116 = for {
                  tunnel: w384 -> [w394] mode=indexing
                  tunnel: [w393] -> w383 mode=indexing
                  n117 = Cluster To Array(cluster=w394) -> (array=w393:string[])
                }
              }
              frame True {
                n118 = for {
                  shift-right: [w429] -> w404
                  shift-left: w409 -> [w428]
                  tunnel: w406 -> [w420] mode=indexing
                  tunnel: w408 -> [w422]
                  tunnel: w407 -> [w421]
                  tunnel: w405 -> [w427]
                  tunnel: [w421] -> w400
                  tunnel: [w422] -> w399
                  w417 = "NULL"
                  n119 = local read "PRODUCE_data_ctr"() -> (w426:refnum<vi>[])
                  n120 = Insert Into Array(array=w420, index=0, new element=string[] []) -> (w413:string[])
                  n121 = Index Array(array=w413, index=7) -> (element=w411:string)
                  n122 = Replace Array Subset(array=w413, new element=w411, index=9) -> (w410:string[])
                  n123 = for {
                    tunnel: w410 -> [w436] mode=indexing
                    tunnel: w426 -> [w441]
                    tunnel: [w435] -> w423
                    i -> [w434]
                    n124 = Add(x=w434, y=2) -> (x+y=w438:i32)
                    n125 = In Range and Coerce(upper limit=11, x=w434, lower limit=7) -> (In Range?=w431:bool)  [unwired: 1 out]
                    n126 = case shown="True" w431 {
                      tunnel: [w442 w446] -> w437
                      tunnel: w436 -> [w444 w445]
                      frame True {
                        n127 = Decimal String To Number(string=w444) -> (number=w443:i32)  [unwired: 2 in, 1 out]
                        n128 = To Variant(anything=w443) -> (Variant=w442:variant)
                      }
                      frame False {
                        n129 = To Variant(anything=w445) -> (Variant=w446:variant)
                      }
                    }
                    n130 = Index Array(array=w441, index=w438) -> (element=w440:refnum<vi>)
                    n131 = property class="Ctl"(reference=w440, "Value"=w437) -> (error out=w435:errorcluster)  [unwired: 1 in, 1 out]
                  }
                  n132 = local read "ECODE"() -> (w416:string)
                  n133 = property on="produce_data" class="Clust (strict)"(error in=w423) -> ("Value"=w425:T1)  [unwired: 1 in, 2 out]
                  n134 = local read "PRODUCE_data_name"() -> (w415:string[])
                  n135 = Bundle By Name(cluster=w425, "PRODUCE_TIME"=w421, "PRODUCE_CODE"=w422, "ITEM_NO"=w417, "LOT_MAKER"=w417, "RETURN_MAN"=w417, "EXPORT_MAN"=w416) -> (w424:T1)
                  "output cluster" <- w424
                  n136 = To Variant(anything=w424) -> (Variant=w430:variant)
                  n137 = call <vilib>:"DB Tools Insert Data.vi"("data"=w430, "columns"=w415, "table"=w427, "connection reference"=w428) -> ("connection reference out"=w429:T4)  [unwired: 6 in, 1 out]
                }
                n138 = Bundle("date/time string"=w400, "produce Code"=w399) -> (w398:T15)  [unwired: 1 in]
                n139 = To Variant(anything=w398) -> (Variant=w397:variant)
                n140 = call <vilib>:"DB Tools Insert Data.vi"("data"=w397, "columns"=string[] ["TIME", "INVOICE_CODE"], "table"=w402, "connection reference"=w404) -> ("connection reference out"=w403:T4)  [unwired: 6 in, 1 out]
              }
            }
            n141 = Index Array(array=w362, index (col)=4 ("disabled index (col)")) -> (element=w360:string[])  [unwired: 1 in]
            n142 = property on="Part No (F2)" class="CmbBox"("Strings[]"=w360) -> ()  [unwired: 2 in, 2 out]
          }
          event "Barcode (F1)": Value Change {
            w494 = 7  # Part No
            w513 = 1  # Barcode
            w516 = 0  # Lot maker
            # "?"
            # "D"
            # "PART NO=MAKER CODE"
            # ".item_information"
            n143 = event-data() -> ("NewVal"=w522:string)  [unwired: 1 in]
            n144 = local read "Length"() -> (w518:string)
            n145 = local read "reference"() -> (w492:refnum<vi>[])
            n146 = To Upper Case(1:w522) -> (0:w517:string)
            n147 = case shown="\"\", \"0\"" w518 {
              selector: w518 -> [_ w531]
              tunnel: w517 -> [w529 w535]
              tunnel: [w529 w534] -> w500
              frame "", "0" {
              }
              frame "1", Default {
                n148 = local read "Offset"() -> (w533:string)
                n149 = Decimal String To Number(string=w533) -> (number=w532:i32)  [unwired: 2 in, 1 out]
                n150 = Decimal String To Number(string=w531) -> (number=w530:i32)  [unwired: 2 in, 1 out]
                n151 = String Subset(string=w535, offset (0)=w532, length (rest)=w530) -> (substring=w534:string)
              }
            }
            n152 = Index Array(array=w492, index #1=w516, index #2=w513, index #3=w494) -> (element #1=w495:refnum<vi>, element #2=w496:refnum<vi>, element #3=w493:refnum<vi>)
            n153 = local read "Product"() -> (w525:string)
            n154 = local read "Part Name"() -> (w524:string)
            n155 = local read "Maker"() -> (w523:string)
            n156 = invoke class="Ctl" method="Reinit To Default"(reference=w493) -> ()  [unwired: 2 in, 3 out]
            n157 = Format Into String(format string="where PRODUCT='%s' \nand PART_NAME='%s' \nand MAKER='%s' \nand (PART_NO ='%s'\nor BARCODE ='%s')", w525, w524, w523, w500, w500) -> (resulting string=w497:string)  [unwired: 2 in, 1 out]
            n158 = call <vilib>:"DB Tools Select Data.vi"("condition"=w497, "columns"=string[] ["ITEM_CODE", "LOT_SIZE", "UNIT", "INVENTORY_LOCAL", "PART_NO"], "table"=w514, "connection reference"=w528) -> ("data"=w521:variant[][], "connection reference out"=w501:T4)  [unwired: 2 in, 1 out]
            n159 = xnode "Database Variant To Data"("database variant"=w521, "type"=string[][] []) -> ("data"=w511:string[][])  [unwired: 1 in, 1 out]
            n160 = Empty Array?(array=w511) -> (empty?=w519:bool)
            n161 = case shown="False" w519 {
              tunnel: w511 -> [w581 _]
              tunnel: [w541 _] -> w509
              tunnel: w511 -> [w577 _]
              tunnel: w510 -> [w576 _]
              tunnel: [w575 w640] -> w508
              tunnel: w507 -> [_ w640]
              tunnel: [w574 w639] -> w506
              tunnel: w505 -> [_ w639]
              tunnel: w502 -> [w539 w637]
              tunnel: w501 -> [w573 w638]
              tunnel: [w537 w638] -> w498
              tunnel: w499 -> [w555 _]
              tunnel: w492 -> [w543 _]
              tunnel: [w538 w637] -> w491
              frame False {
                w547 = 0 ("index (row)")
                w566 = 0 ("index (row)")
                w580 = 1  # Item code
                # "?"
                # "hien thi tren cung"
                # "co the tim trong  table hay khong ?"
                # "quet va tim trong array file, co thi xuat ra row data"
                # ".iqa"
                # "chua co thi tao bang new_item trong warehouse_database"
                n162 = for {
                  tunnel: w581 -> [w629] mode=indexing
                  n163 = for {
                    tunnel: w629 -> [w630] mode=indexing
                    i -> [w631]
                    n164 = case shown="1" w631 {
                      tunnel: w630 -> [w632 w633 w634 w635 w636 _]
                      frame 0 {
                        n165 = local write "Item Code (F3)"(w632) -> ()
                      }
                      frame 1 {
                        n166 = local write "Lot Size (F6)"(w633) -> ()
                      }
                      frame 2 {
                        n167 = local write "Unit (F7)"(w634) -> ()
                      }
                      frame 3 {
                        n168 = local write "Location (F5)"(w635) -> ()
                      }
                      frame 4 {
                        n169 = local write "Maker Code (F4)"(w636) -> ()
                      }
                      frame 5, Default {
                      }
                    }
                  }
                }
                n170 = Index Array(array=w577, index (row) #1=w566, index (col) #1=w566, index (row) #2=w566, index (col) #2=3 ("disabled index (col)")) -> (element #1=w556:string, element #2=w571:string)
                n171 = Empty String/Path?(string/path=w571) -> (empty?=w572:bool)
                n172 = call "Search element.vi"("element"=w556, "Colum"=w580, "all data"=w576) -> ("row data"=w575:string[], "Status"=w541:bool, "index"=w574:i32)  [unwired: 5 in, 1 out]
                n173 = Select(t="new_item", s=w572, f=w571) -> (s? t:f=w563:string)
                n174 = To Lower Case(string=w563) -> (all lower case string=w562:string)
                n175 = Bundle("index"=w574, 0) -> (w578:cluster{"index":i32, i32})  [unwired: 1 in]
                n176 = property on="Table" class="Tbl (strict)"("Index Values"=w578) -> ()  [unwired: 2 in, 2 out]
                n177 = Format Into String(format string="`warehouse_database`.`%s`", w562) -> (resulting string=w564:string)  [unwired: 2 in, 1 out]
                "stock" <- w564
                n178 = Format Into String(format string="CREATE TABLE %s(\n`ITEM_CODE` VARCHAR(30) NOT NULL,\n`INVOICE_DATE` VARCHAR(30) NOT NULL, \n`INVOICE_NO` VARCHAR(45) NOT NULL, \n`QUANTITY` VARCHAR(10) NOT NULL, \n`LOT_MAKER` VARCHAR(255) NOT NULL,  \n`ITEM_NO` VARCHAR(6) NOT NULL,\n`IQA` VARCHAR(5) NULL,\n`WAREHOUSE` VARCHAR(10) NULL,\nPRIMARY KEY (`ITEM_CODE`,`INVOICE_NO`,`ITEM_NO`))", w564) -> (resulting string=w568:string)  [unwired: 2 in, 1 out]
                n179 = call "Creat table.vi"("query"=w568, "table name"=w562, "table data"=w539, "Refnum in"=w573) -> ("table data"=w538:string[], "Refnum out"=w557:T4)  [unwired: 6 in]
                n180 = local read "produce Code"() -> (w561:string)
                n181 = Format Into String(format string="where INVOICE_CODE='%s' \nand ITEM_CODE='%s'; ", w561, w556) -> (resulting string=w560:string)  [unwired: 2 in, 1 out]
                n182 = call <vilib>:"DB Tools Select Data.vi"("condition"=w560, "columns"=string[] ["ITEM_NO", "BALANCE", "IQA"], "table"=w555, "connection reference"=w557) -> ("data"=w544:variant[][], "connection reference out"=w537:T4)  [unwired: 2 in, 1 out]
                n183 = xnode "Database Variant To Data"("database variant"=w544, "type"=string[][] []) -> ("data"=w553:string[][])  [unwired: 1 in, 1 out]
                n184 = Index Array(array=w553, index (row) #1=w547, index (col) #1=w547, index (row) #2=w547, index (col) #2=1 ("index (row)"), index (row) #3=w547, index (col) #3=2 ("index (row)")) -> (element #1=w552:string, element #2=w550:string, element #3=→"IQA":string)
                n185 = Decimal String To Number(string=w552) -> (number=w540:i32)  [unwired: 2 in, 1 out]
                n186 = Decimal String To Number(string=w550) -> (number=w549:i32)  [unwired: 2 in, 1 out]
                n187 = Equal To 0?(x=w549) -> (x = 0?=w548:bool)
                n188 = Increment(x=w540) -> (x+1=w536:i32)
                n189 = And(x=w548, y=w541) -> (x .and. y?=w542:bool)
                n190 = local write "Item No.(F8)"(w536) -> ()
                n191 = case shown="True" w542 {
                  tunnel: w543 -> [_ w582]
                  frame False {
                  }
                  frame True {
                    n192 = for {
                      tunnel: w582 -> [w584] mode=indexing
                      n193 = invoke class="Ctl" method="Reinit To Default"(reference=w584) -> ()  [unwired: 2 in, 3 out]
                    }
                    n194 = One Button Dialog(message="Quantity is Enough!") -> ()  [unwired: 1 in, 1 out]
                  }
                }
              }
              frame True {
                n195 = One Button Dialog(message="THIS ITEM DON'T HAVE INFORMATION.\nPLEASE ADD INFORMATION !", button name ("OK")="OK") -> ()  [unwired: 1 out]
              }
            }
            n196 = Select(t=w495, s=w509, f=w496) -> (s? t:f=w512:refnum<vi>)
            n197 = property class="Ctl"(reference=w512, "Key Focus"=TRUE) -> ()  [unwired: 1 in, 2 out]
          }
          event "Barcode (F1)", "Part No (F2)": Mouse Up {
            n198 = event-data() -> ()  [unwired: 1 in, 8 out]
            n199 = local read "reference"() -> (w694:refnum<vi>[])
            n200 = for {
              tunnel: w694 -> [w695] mode=indexing
              n201 = invoke class="Ctl" method="Reinit To Default"(reference=w695) -> ()  [unwired: 2 in, 3 out]
            }
          }
          event "Part No (F2)": Value Change {
            w697 = 7  # Part No
            w717 = 1  # Barcode
            w720 = 0  # Lot maker
            n202 = event-data() -> ("NewVal"=w724:string)  [unwired: 1 in]
            n203 = local read "reference"() -> (w698:refnum<vi>[])
            n204 = To Upper Case(1:w724) -> (0:w700:string)
            n205 = local read "Product"() -> (w727:string)
            n206 = local read "Part Name"() -> (w726:string)
            n207 = local read "Maker"() -> (w725:string)
            n208 = Index Array(array=w698, index #1=w720, index #2=w717, index #3=w697) -> (element #1=w701:refnum<vi>, element #2=w699:refnum<vi>)  [unwired: 1 out]
            n209 = Format Into String(format string="where PRODUCT='%s' \nand PART_NAME='%s' \nand MAKER='%s' \nand PART_NO ='%s'", w727, w726, w725, w700) -> (resulting string=w702:string)  [unwired: 2 in, 1 out]
            n210 = invoke class="Ctl" method="Reinit To Default"(reference=w699) -> ()  [unwired: 2 in, 3 out]
            n211 = call <vilib>:"DB Tools Select Data.vi"("condition"=w702, "columns"=string[] ["ITEM_CODE", "LOT_SIZE", "UNIT", "INVENTORY_LOCAL", "PART_NO"], "table"=w718, "connection reference"=w730) -> ("data"=w723:variant[][], "connection reference out"=w705:T4)  [unwired: 2 in, 1 out]
            n212 = xnode "Database Variant To Data"("database variant"=w723, "type"=string[][] []) -> ("data"=w715:string[][])  [unwired: 1 in, 1 out]
            n213 = Empty Array?(array=w715) -> (empty?=w721:bool)
            n214 = case shown="False" w721 {
              tunnel: w715 -> [w776 _]
              tunnel: [w737 _] -> w713
              tunnel: w715 -> [w772 _]
              tunnel: w714 -> [w771 _]
              tunnel: [w770 w835] -> w712
              tunnel: w711 -> [_ w835]
              tunnel: [w769 w834] -> w710
              tunnel: w709 -> [_ w834]
              tunnel: w706 -> [w732 w832]
              tunnel: w705 -> [w768 w833]
              tunnel: [w739 w833] -> w703
              tunnel: w704 -> [w751 _]
              tunnel: w698 -> [w740 _]
              tunnel: [w731 w832] -> w696
              frame False {
                w743 = 0 ("index (row)")
                w761 = 0 ("index (row)")
                w775 = 1  # Item code
                # "? GIONG VOI BARCODE CHANGE VALUE"
                n215 = for {
                  tunnel: w776 -> [w824] mode=indexing
                  n216 = for {
                    tunnel: w824 -> [w825] mode=indexing
                    i -> [w826]
                    n217 = case shown="4" w826 {
                      tunnel: w825 -> [w827 w828 w829 w830 w831 _]
                      frame 0 {
                        n218 = local write "Item Code (F3)"(w827) -> ()
                      }
                      frame 1 {
                        n219 = local write "Lot Size (F6)"(w828) -> ()
                      }
                      frame 2 {
                        n220 = local write "Unit (F7)"(w829) -> ()
                      }
                      frame 3 {
                        n221 = local write "Location (F5)"(w830) -> ()
                      }
                      frame 4 {
                        n222 = local write "Maker Code (F4)"(w831) -> ()
                      }
                      frame 5, Default {
                      }
                    }
                  }
                }
                n223 = Index Array(array=w772, index (row) #1=w761, index (col) #1=w761, index (row) #2=w761, index (col) #2=3 ("disabled index (col)")) -> (element #1=w752:string, element #2=w766:string)
                n224 = Empty String/Path?(string/path=w766) -> (empty?=w767:bool)
                n225 = call "Search element.vi"("element"=w752, "Colum"=w775, "all data"=w771) -> ("row data"=w770:string[], "Status"=w737:bool, "index"=w769:i32)  [unwired: 5 in, 1 out]
                n226 = Select(t="new_item", s=w767, f=w766) -> (s? t:f=w759:string)
                n227 = To Lower Case(string=w759) -> (all lower case string=w758:string)
                n228 = Bundle("index"=w769, 0) -> (w773:cluster{"index":i32, i32})  [unwired: 1 in]
                n229 = property on="Table" class="Tbl (strict)"("Index Values"=w773) -> ()  [unwired: 2 in, 2 out]
                n230 = Format Into String(format string="`warehouse_database`.`%s`", w758) -> (resulting string=w734:string)  [unwired: 2 in, 1 out]
                n231 = local write "stock"(w734) -> ()
                n232 = Format Into String(format string="CREATE TABLE %s(\n`ITEM_CODE` VARCHAR(30) NOT NULL,\n`INVOICE_DATE` VARCHAR(30) NOT NULL, \n`INVOICE_NO` VARCHAR(45) NOT NULL, \n`QUANTITY` VARCHAR(10) NOT NULL, \n`LOT_MAKER` VARCHAR(255) NOT NULL,  \n`ITEM_NO` VARCHAR(6) NOT NULL,\n `IQA` VARCHAR(5) NULL,\n`WAREHOUSE` VARCHAR(10) NULL,\nPRIMARY KEY (`ITEM_CODE`,`INVOICE_NO`,`ITEM_NO`))", w734) -> (resulting string=w763:string)  [unwired: 2 in, 1 out]
                n233 = call "Creat table.vi"("query"=w763, "table name"=w758, "table data"=w732, "Refnum in"=w768) -> ("table data"=w731:string[], "Refnum out"=w753:T4)  [unwired: 6 in]
                n234 = local read "produce Code"() -> (w757:string)
                n235 = Format Into String(format string="where INVOICE_CODE='%s' \nand ITEM_CODE='%s'; ", w757, w752) -> (resulting string=w756:string)  [unwired: 2 in, 1 out]
                n236 = call <vilib>:"DB Tools Select Data.vi"("condition"=w756, "columns"=string[] ["ITEM_NO", "BALANCE", "IQA"], "table"=w751, "connection reference"=w753) -> ("data"=w741:variant[][], "connection reference out"=w739:T4)  [unwired: 2 in, 1 out]
                n237 = xnode "Database Variant To Data"("database variant"=w741, "type"=string[][] []) -> ("data"=w749:string[][])  [unwired: 1 in, 1 out]
                n238 = Index Array(array=w749, index (row) #1=w743, index (col) #1=w743, index (row) #2=w743, index (col) #2=1 ("index (row)"), index (row) #3=w743, index (col) #3=2 ("index (row)")) -> (element #1=w748:string, element #2=w746:string, element #3=w735:string)
                n239 = local write "IQA"(w735) -> ()
                n240 = Decimal String To Number(string=w748) -> (number=w736:i32)  [unwired: 2 in, 1 out]
                n241 = Decimal String To Number(string=w746) -> (number=w745:i32)  [unwired: 2 in, 1 out]
                n242 = Equal To 0?(x=w745) -> (x = 0?=w744:bool)
                n243 = Increment(x=w736) -> (x+1=w733:i32)
                n244 = And(x=w744, y=w737) -> (x .and. y?=w738:bool)
                n245 = local write "Item No.(F8)"(w733) -> ()
                n246 = case shown="True" w738 {
                  tunnel: w740 -> [_ w777]
                  frame False {
                  }
                  frame True {
                    n247 = for {
                      tunnel: w777 -> [w779] mode=indexing
                      n248 = invoke class="Ctl" method="Reinit To Default"(reference=w779) -> ()  [unwired: 2 in, 3 out]
                    }
                    n249 = One Button Dialog(message="Quantity is Enough!") -> ()  [unwired: 1 in, 1 out]
                  }
                }
              }
              frame True {
                n250 = One Button Dialog(message="THIS ITEM DON'T HAVE INFORMATION.\nPLEASE ADD INFORMATION !", button name ("OK")="OK") -> ()  [unwired: 1 out]
              }
            }
            n251 = Select(t=w701, s=w713, f=w699) -> (s? t:f=w716:refnum<vi>)
            n252 = property class="Ctl"(reference=w716, "Key Focus"=TRUE) -> ()  [unwired: 1 in, 2 out]
          }
          event "BUTTON_ADD": Value Change {
            # ".item_information"
            n253 = event-data() -> ()  [unwired: 1 in, 1 out]
            n254 = local read "Item Code (F3)"() -> (w897:string)
            n255 = local read "Length"() -> (w888:string)
            n256 = local read "Offset"() -> (w890:string)
            n257 = local read "Barcode (F1)"() -> (w892:string)
            n258 = Format Into String(format string="where ITEM_CODE='%s';" ("condition"), w897) -> (resulting string=w885:string)  [unwired: 2 in, 1 out]
            n259 = To Upper Case(1:w892) -> (0:w889:string)
            n260 = call <vilib>:"DB Tools Select Data.vi"("condition"=w885, "columns"=string[] ["PART_NO"], "table"=w900, "connection reference"=w902) -> ("data"=w896:variant[][], "connection reference out"=w901:T4)  [unwired: 2 in, 1 out]
            n261 = Concatenate Strings "Concatenate Strings"(w888, "-" ("string"), w890) -> (w886:string)
            n262 = xnode "Database Variant To Data"("database variant"=w896, "type"=string[][] []) -> ("data"=w894:string[][])  [unwired: 1 in, 1 out]
            n263 = Empty Array?(array=w894) -> (empty?=w893:bool)
            n264 = case shown="\"\", \"0\"" w888 {
              selector: w888 -> [_ w909]
              tunnel: w889 -> [w907 w913]
              tunnel: [w907 w912] -> w887
              frame "", "0" {
              }
              frame "1", Default {
                n265 = local read "Offset"() -> (w911:string)
                n266 = Decimal String To Number(string=w911) -> (number=w910:i32)  [unwired: 2 in, 1 out]
                n267 = Decimal String To Number(string=w909) -> (number=w908:i32)  [unwired: 2 in, 1 out]
                n268 = String Subset(string=w913, offset (0)=w910, length (rest)=w908) -> (substring=w912:string)
              }
            }
            n269 = case shown="True" w893 {
              tunnel: [w914 w937] -> w906
              tunnel: w901 -> [w922 w927]
              tunnel: w900 -> [w921 w926]
              tunnel: w897 -> [_ w925]
              tunnel: w887 -> [w918 w923]
              tunnel: w886 -> [w919 w924]
              tunnel: w885 -> [w915 _]
              frame False {
                n270 = Bundle(w919, w918) -> (w917:cluster{string, string})  [unwired: 1 in]
                n271 = To Variant(anything=w917) -> (Variant=w916:variant)
                n272 = call <vilib>:"DB Tools Update Data.vi"("condition"=w915, "data"=w916, "columns"=string[] ["`LENGTH-OFFSET`", "BARCODE"], "table"=w921, "connection reference"=w922) -> ("connection reference out"=w914:T4)  [unwired: 5 in, 1 out]
              }
              frame True {
                # "THEM DU LIEU VAO BANG item_information"
                n273 = local read "Maker Code (F4)"() -> (w932:string)
                n274 = local read "Lot Size (F6)"() -> (w936:string)
                n275 = local read "Unit (F7)"() -> (w931:string)
                n276 = local read "Location (F5)"() -> (w930:string)
                n277 = local read "Part Name"() -> (w934:string)
                n278 = local read "Maker"() -> (w933:string)
                n279 = local read "Product"() -> (w935:string)
                n280 = Bundle("Product"=w935, "Item Code (F3)"=w925, "Part Name"=w934, "Maker"=w933, "Maker Code (F4)"=w932, "Lot Size (F6)"=w936, "Unit (F7)"=w931, w924, w923, "Location (F5)"=w930) -> (w929:T16)  [unwired: 1 in]
                n281 = To Variant(anything=w929) -> (Variant=w928:variant)
                n282 = call <vilib>:"DB Tools Insert Data.vi"("data"=w928, "columns"=string[] ["PRODUCT", "ITEM_CODE", "PART_NAME", "MAKER", "PART_NO", "LOT_SIZE", "UNIT", "`LENGTH-OFFSET`", "BARCODE", "INVENTORY_LOCAL"], "table"=w926, "connection reference"=w927) -> ("connection reference out"=w937:T4)  [unwired: 6 in, 1 out]
              }
            }
          }
          event "Print": Value Change {
            n283 = event-data() -> ()  [unwired: 1 in, 1 out]
            n284 = local read "Maker Code (F4)"() -> (w996:string)
            n285 = local read "Item Code (F3)"() -> (w997:string)
            n286 = local read "Quantity (F10)"() -> (w994:string)
            n287 = local read "Lot Maker (F9)"() -> (w986:string)
            n288 = local read "Product"() -> (w993:string)
            n289 = local read "Maker"() -> (w995:string)
            n290 = Empty String/Path?(string/path=w997) -> (empty?=w992:bool)
            n291 = Empty String/Path?(string/path=w996) -> (empty?=w991:bool)
            n292 = Empty String/Path?(string/path=w995) -> (empty?=w990:bool)
            n293 = Empty String/Path?(string/path=w994) -> (empty?=w989:bool)
            n294 = Empty String/Path?(string/path=w993) -> (empty?=w988:bool)
            n295 = Empty String/Path?(string/path=w986) -> (empty?=w985:bool)
            n296 = Compound Arithmetic op=OR(w992, w991, w990, w989, w988, w985) -> (w987:bool)
            n297 = case shown="False" w987 {
              tunnel: w1006 -> [w1038 _]
              tunnel: w1005 -> [w1036 w1091]
              tunnel: [w1024 w1091] -> w1003
              tunnel: w1002 -> [w1023 w1090]
              tunnel: [w1022 w1090] -> w1001
              tunnel: w1000 -> [w1021 _]
              tunnel: w999 -> [w1020 _]
              tunnel: w998 -> [w1018 _]
              tunnel: w984 -> [w1013 _]
              frame False {
                # "chen vao bang stock"
                n298 = local read "Produce Date"() -> (w1016:timestamp)
                n299 = local read "Item No.(F8)"() -> (w1011:i32)
                n300 = Format Date/Time String(time format string (%c)="%d/%m/%Y", seconds (now)=w1016) -> (date/time string=w1015:string)  [unwired: 1 in]
                n301 = case shown="True" "Print Mode" {
                  tunnel: w1036 -> [w1058 w1081]
                  tunnel: [w1058 w1075] -> w1024
                  tunnel: w1023 -> [w1057 w1074]
                  tunnel: [w1057 w1073] -> w1022
                  tunnel: w1021 -> [_ w1072]
                  tunnel: w1020 -> [_ w1071]
                  tunnel: [_ w1070] -> w1019
                  tunnel: w1018 -> [_ w1069]
                  tunnel: w1015 -> [_ w1065]
                  tunnel: w1011 -> [w1056 w1063]
                  tunnel: w1013 -> [_ w1064]
                  tunnel: [w1055 w1062] -> w1012
                  frame False {
                    n302 = Number To Decimal String(number=w1056) -> (decimal integer string=w1055:string)  [unwired: 1 in]
                  }
                  frame True {
                    n303 = Number To Decimal String(number=w1063) -> (decimal integer string=w1062:string)  [unwired: 1 in]
                    n304 = local read "item_data"() -> (w1068:T2)
                    n305 = local read "item_data_name"() -> (w1067:string[])
                    n306 = local read "stock"() -> (w1061:string)
                    n307 = local read "produce Code"() -> (w1078:string)
                    n308 = local read "IQA"() -> (w1060:string)
                    n309 = local read "Lot Maker (F9)"() -> (w1076:string)
                    n310 = local read "Item Code (F3)"() -> (w1077:string)
                    n311 = local read "Quantity (F10)"() -> (w1080:string)
                    n312 = local read "ECODE"() -> (w1079:string)
                    n313 = Bundle("Quantity (F10)"=w1080, "ECODE"=w1079, "produce Code"=w1078, "Item Code (F3)"=w1077, "Lot Maker (F9)"=w1076, "stock"=w1061, "IQA"=w1060, "") -> (w1066:T17)  [unwired: 1 in]
                    n314 = call "Import Invoice data.vi"("Refnum in"=w1081, "iqa"=w1069, "item_data"=w1068, "item_data_name"=w1067, "Invoive date"=w1065, "Item no"=w1062, "File data in"=w1074, "Import Data"=w1066, "row data"=w1072, "index"=w1071, "item"=w1064) -> ("Refnum out"=w1075:T4, "File data out"=w1073:string[][], "error out"=w1070:errorcluster)  [unwired: 6 in]
                  }
                }
                n315 = disable-structure shown="Enabled" {
                  disable-tunnel: [path "G:/06. Data/Data/05. AEC/07. New Storage Management/Setting/LABEL.xlsx" ("template (empty)") w1083] -> w1035
                  frame Disabled {
                    # "caution"
                  }
                  frame Enabled {
                    n316 = Build Path(base path="Path", name or relative path="Setting") -> (appended path=w1085:path)
                    n317 = Build Path(base path=w1085, name or relative path="LABEL.xlsx") -> (appended path=w1083:path)
                  }
                }
                n318 = local read "Maker Code (F4)"() -> (w1032:string)
                n319 = local read "Item Code (F3)"() -> (w1034:string)
                n320 = local read "Lot Maker (F9)"() -> (w1026:string)
                n321 = local read "Quantity (F10)"() -> (w1030:string)
                n322 = local read "produce Code"() -> (w1027:string)
                n323 = local read "Location (F5)"() -> (w1029:string)
                n324 = local read "Unit (F7)"() -> (w1025:string)
                n325 = local read "Product"() -> (w1028:string)
                n326 = local read "ECODE"() -> (w1033:string)
                n327 = local read "Maker"() -> (w1031:string)
                n328 = Bundle By Name(cluster=T11 {"Item Code"="", "ECode"="", "Part No."="", "Maker"="", "Quantity"="", "Location"="", "Product"="", "Invoice No"="", "Invoice Date"="", "Lot maker"="", "Item No"="", "Unit"=""} ("Item_Information"), "Item Code"=w1034, "ECode"=w1033, "Part No."=w1032, "Maker"=w1031, "Quantity"=w1030, "Location"=w1029, "Product"=w1028, "Invoice No"=w1027, "Invoice Date"=w1015, "Lot maker"=w1026, "Item No"=w1012, "Unit"=w1025) -> (w1009:T11)
                n329 = call "insert string&image into excel.vi"("error in"=w1019, "Item_Information"=w1009, "template Path"=w1035) -> ("error out"=w1008:errorcluster)  [unwired: 7 in, 1 out]
                n330 = case shown="False" "Print Mode 2" {
                  tunnel: w1038 -> [_ w1045]
                  tunnel: [w1042 w1044] -> w1037
                  tunnel: w1008 -> [w1042 w1043]
                  frame False {
                    n331 = local read "Item No.(F8)"() -> (w1041:i32)
                    n332 = Increment(x=w1041) -> (x+1=w1040:i32)
                    n333 = local write "Item No.(F8)"(w1040) -> ()
                  }
                  frame True {
                    n334 = for {
                      tunnel: w1045 -> [w1048] mode=indexing
                      tunnel: [w1047] -> w1044
                      tunnel: w1043 -> [w1046]
                      i -> [w1051]
                      n335 = Greater Or Equal?(x=w1051, y=9) -> (x >= y?=w1049:bool)
                      n336 = case shown="True" w1049 {
                        tunnel: w1048 -> [_ w1054]
                        tunnel: [_ w1053] -> w1047
                        tunnel: w1046 -> [_ w1052]
                        frame False {
                        }
                        frame True {
                          n337 = invoke class="Ctl" method="Reinit To Default"(reference=w1054, error in=w1052) -> (error out=w1053:errorcluster)  [unwired: 1 in, 2 out]
                        }
                      }
                    }
                  }
                }
                n338 = property on="Barcode (F1)" class="Str"(error in=w1037, "Key Focus"=TRUE) -> ()  [unwired: 1 in, 2 out]
              }
              frame True {
                n339 = One Button Dialog(message="Please check all information!\nITEM CODE\nMAKER CODE\nMAKER\nPRODUCT\nLOT MAKER\nQUANTITY", button name ("OK")="OK") -> ()  [unwired: 1 out]
              }
            }
          }
          event "Maker": Value Change {
            n340 = event-data() -> ("NewVal"=w1095:string)  [unwired: 1 in, 5 out]
            n341 = local read "Part Name"() -> (w1104:string)
            n342 = local read "Product"() -> (w1105:string)
            n343 = Empty String/Path?(string/path=w1105) -> (empty?=w1108:bool)
            n344 = Empty String/Path?(string/path=w1095) -> (empty?=w1094:bool)
            n345 = Empty String/Path?(string/path=w1104) -> (empty?=w1107:bool)
            n346 = Compound Arithmetic op=AND(w1108, w1107, w1094) -> (w1106:bool)
            n347 = case shown="False" w1106 {
              tunnel: w1095 -> [w1120 _]
              tunnel: w1105 -> [w1122 _]
              tunnel: w1104 -> [w1121 _]
              tunnel: w1103 -> [w1115 w1175]
              tunnel: [w1114 w1175] -> w1102
              tunnel: w1100 -> [w1113 _]
              tunnel: w1093 -> [w1109 _]
              frame False {
                w1112 = 9  # Barcode
                n348 = Index Array(array=w1113, index=w1112) -> (element=w1111:refnum<vi>)
                n349 = Format Into String(format string="where PRODUCT='%s'\n and PART_NAME='%s'\n and MAKER='%s'" ("condition"), w1122, w1121, w1120) -> (resulting string=w1130:string)  [unwired: 2 in, 1 out]
                n350 = property class="Ctl"(reference=w1111, "Key Focus"=TRUE) -> ()  [unwired: 1 in, 2 out]
                n351 = call <vilib>:"DB Tools Select Data.vi"("condition"=w1130, "columns"=string[] ["`LENGTH-OFFSET`"], "table"=w1109, "connection reference"=w1115) -> ("data"=w1124:variant[][], "connection reference out"=w1114:T4)  [unwired: 2 in, 1 out]
                n352 = xnode "Database Variant To Data"("database variant"=w1124, "type"=string[][] []) -> ("data"=w1126:string[][])  [unwired: 1 in, 1 out]
                n353 = Index Array(array=w1126, index (row)=0, index (col)=0 ("disabled index (col)")) -> (element=w1119:string)
                n354 = Match Pattern(string=w1119, regular expression="-") -> (before substring=w1117:string, after substring=w1116:string)  [unwired: 1 in, 2 out]
                n355 = local write "Offset"(w1116) -> ()
                n356 = local write "Length"(w1117) -> ()
              }
              frame True {
              }
            }
          }
          event "Lot Maker (F9)": Value Change {
            w1186 = 17  # Quantity
            n357 = event-data() -> ()  [unwired: 1 in, 6 out]
            n358 = local read "Lot Size (F6)"() -> (w1177:string)
            n359 = Index Array(array=w1187, index=w1186) -> (element=w1185:refnum<vi>)
            n360 = property class="Ctl"(reference=w1185, "Key Focus"=TRUE, "Value"=w1177) -> ()  [unwired: 1 in, 2 out]
          }
          event Panel Close? {
            n361 = event-data() -> ()  [unwired: 1 in, 4 out]
            n362 = call "Exit.vi"() -> ("T button?"=w1195:bool)  [unwired: 11 in]
            n363 = Not(x=w1195) -> (.not. x?=w1196:bool)
            n364 = event-data("Discard?"=w1196) -> ()  [unwired: 1 in, 1 out]
          }
        }
        "Table" <- w277
      }
      frame "Exit" {
      }
    }
  }
  n365 = disable-structure shown="Enabled" {
    disable-tunnel: w15 -> [w1202 w1203]
    disable-tunnel: [_ w1203] -> w14
    frame Enabled {
      # "caution"
      n366 = call <vilib>:"DB Tools Close Connection.vi"("connection reference"=w1202) -> ()  [unwired: 6 in, 1 out]
    }
    frame Disabled {
    }
  }
  "connection out" <- w14
